vi "CRYUnflatten Stimulus Element.vi"(8 "error in (no error)":errorcluster, 11 "Unflatten Stimulus Element setup":string) -> (0 "error out":errorcluster, 1 "Stimulus Para":T1={"Name"="", "Level Out"=0.9999999999999998, "Start Freq"=6300.0, "Stop Freq"=100.0, "Steps"=19, "Cycles"=12, "Sweep type"=0, "Freq"=1000.0, "Start ampl"=0.9999999999999998, "Stop ampl"=0.9999999999999998, "sine waves"=[], "wav path"="", "Sweep time"=0.9999999999999998, "Resolution"=0, "Tone type6"=0, "fix/ratio6"=0, "Ratio6"=0, "Difference6"=0, "RatioFreq6"=0} {"Resolution" items=["R10(1/3 Oct.)", "R20(1/6 Oct.)", "R40(1/12 Oct.)", "R80(1/24 Oct.)", "User Defined, Log", "User Defined,Linear"]; "Sweep time" format="%.2f"; "Stop ampl" format="%.2f"; "Start ampl" format="%.2f"; "Freq" format="%.2f"; "sine waves"."cycles" format="%.2f"; "sine waves"."ampl" format="%.2f"; "sine waves"."freq" format="%.2f"; "Level Out" format="%.2f"}, 2 "Stimulus Default":T10={"fstepsw"={"Level(U)"=1.0, "Start Freq(Hz)"=6300.0, "Stop Freq(Hz)"=100.0, "ML val level name"="", "Use ML Val level?"=FALSE, "ML axis"=1, "Steps (#)"=19, "Cycles/step(#)"=8, "Time/step (s)"=0.01, "Step Resolution"=0, "unit"=0, "Start Freq Name"="", "Stop Freq Name"="", "Start Freq Axis"=1, "Stop Freq Axis"=1, "Start Freq Flag"="", "Stop Freq Flag"="", "Output Imp"=6300.0, "Nominal Imp"=100.0, "V on DUT"=FALSE}, "flogsw"={"Level(U)"=1.0, "Start Freq(Hz)"=100.0, "Stop Freq(Hz)"=6300.0, "Sweep Rate(s/dec)"=1.0, "Use ML Val level?"=FALSE, "ML val level name"="", "ML axis"=1, "TSR params"={"FSamp"=0.0, "FStart"=0.0, "FStop"=0.0, "NOffset"=0.0, "MStop"=0.0, "MStart"=0.0, "NHarm"=0.0, "Tsamp"=0.0, "Amplit"=0.0}, "unit"=0, "Start Freq Name"="", "Stop Freq Name"="", "Start Freq Axis"=1, "Stop Freq Axis"=1, "Start Freq Flag"="", "Stop Freq Flag"="", "Output Imp"=6300.0, "Nominal Imp"=100.0, "V on DUT"=FALSE}, "ampsw"={"Freq(Hz)"=1000.0, "Steps (#)"=19, "Cycles(#)"=12, "Use ML Val freq?"=FALSE, "ML val freq name"="", "ML axis"=1, "Start Ampl(U)"=0.5, "Stop Ampl(U)"=1.0, "unit"=0}, "wavefile"={"Level(U)"=0.0, "Wave Path"="", "ML axis"=1, "ML val level name"="", "Use ML Val level?"=FALSE, "wave info"="", "wave time"="", "Peak value4"=0.0, "RMS value4"=0.0, "wave channel"=0, "unit"=0, "Output Imp"=6300.0, "Nominal Imp"=100.0, "V on DUT"=FALSE}, "dcconn"={"dc ctrl"=0, "dcmax I"=0, "dc polar"=0, "dc ctrl"=0, "Steps (#)"=19, "Time/step (s)"=0.05, "Start Ampl(U)"=1.0, "Stop Ampl(U)"=1.0, "Level(U)"=1.0, "Step Size"=1.0}, "twotone"={"Steps (#)"=19, "Tone Type"=0, "Freq2(Hz)"=1000.0, "Time/step (s)"=0.0, "Cycles/step (#)"=12, "ML val level name"="", "Use ML Val level?"=FALSE, "Level(U) 2"=1.0, "Diff Freq(Hz)"=100.0, "ML axis 2"=1, "Diff/Ratio"=0, "Level(U)"=1.0, "Stop Freq(Hz)"=100.0, "Ratio Val"=0.8, "ML val level name 2"="", "Use ML Val level? 2"=FALSE, "ML axis"=1, "Start Freq(Hz)"=6300.0, "Step Resolution"=0, "Ratio"=0, "TabCtrl6"=enum."Master Tone", "unit 1"=0, "unit 2"=0, "Start Freq Name"="", "Stop Freq Name"="", "Start Freq Axis"=1, "Stop Freq Axis"=1, "Start Freq Flag"="", "Stop Freq Flag"=""}, "mltitone"={"Level(U)"=0.0, "Min Freq(Hz)"=0.0, "Max Freq(Hz)"=0.0, "Duration(s)"=0.0, "Freq Rounding"=FALSE, "Rounding Val"=5.0, "Profile"=0, "ML axis 2"=0, "ML val level name"="", "Use ML Val level?"=FALSE, "ML axis"=0, "Step Resolution"=0, "unit"=0, "Start Freq Name"="", "Stop Freq Name"="", "Start Freq Axis"=1, "Stop Freq Axis"=1, "Start Freq Flag"="", "Stop Freq Flag"="", "Output Imp"=6300.0, "Nominal Imp"=100.0, "V on DUT"=FALSE}, "noise"={"Noise Type"=0, "Min Freq(Hz)"=20.0, "Max Freq(Hz)"=20000.0, "Level(U)"=1.0, "Duration(s)"=1.0, "ML val level name"="", "Use ML Val level?"=FALSE, "ML axis"=1, "unit"=0, "Start Freq Name"="", "Stop Freq Name"="", "Start Freq Axis"=1, "Stop Freq Axis"=1, "Start Freq Flag"="", "Stop Freq Flag"="", "Output Imp"=6300.0, "Nominal Imp"=100.0, "V on DUT"=FALSE}, "sqwvsw"={"Level(U)"=1.0, "Duty Cycle"=0.0, "ML val level name"="", "ML axis"=1, "Start Freq(Hz)"=6300, "Stop Freq(Hz)"=100, "Use ML Val level?"=FALSE, "Steps (#)"=19, "Cycles/step (#)"=12, "Time/step (s)"=0.0, "Step Resolution"=0}, "tnbrst"={"Level(U)"=1.0, "ML val level name"="", "ML axis"=1, "Start Freq(Hz)"=6300, "Use ML Val level?"=FALSE, "Cycles/step (#)"=12, "Duration(s)"=12.0}} {"tnbrst"."Duration(s)" format="%_2f"; "tnbrst"."Level(U)" format="%_2f"; "sqwvsw"."Step Resolution" items=["R10(1/3 Oct.)", "R20(1/6 Oct.)", "R40(1/12 Oct.)", "R80(1/24 Oct.)", "User Defined, Log", "User Defined,Linear"]; "sqwvsw"."Duty Cycle" format="%_2f"; "sqwvsw"."Level(U)" format="%_2f"; "noise"."Nominal Imp" format="%.2p"; "noise"."Output Imp" format="%.2p"; "noise"."unit" items=["V  RMS", "dB re 1.0 V"]; "noise"."Duration(s)" format="%_2f"; "noise"."Level(U)" format="%_2f"; "mltitone"."Nominal Imp" format="%.2p"; "mltitone"."Output Imp" format="%.2p"; "mltitone"."unit" items=["V  RMS", "dB re 1.0 V"]; "mltitone"."Step Resolution" items=["R10(1/3 Oct.)", "R20(1/6 Oct.)", "R40(1/12 Oct.)", "R80(1/24 Oct.)", "User Defined, Log", "User Defined,Linear"]; "mltitone"."Duration(s)" format="%_2f"; "mltitone"."Level(U)" format="%_2f"; "twotone"."unit 2" items=["V  RMS", "dB re 1.0 V"]; "twotone"."unit 1" items=["V  RMS", "dB re 1.0 V"]; "twotone"."Ratio" items=["R10(1/3 Oct.)", "R20(1/6 Oct.)", "R40(1/12 Oct.)", "R80(1/24 Oct.)", "User Defined, Log", "User Defined,Linear"]; "twotone"."Step Resolution" items=["R10(1/3 Oct.)", "R20(1/6 Oct.)", "R40(1/12 Oct.)", "R80(1/24 Oct.)", "User Defined, Log", "User Defined,Linear"]; "twotone"."Ratio Val" format="%_2f"; "twotone"."Level(U)" format="%_2f"; "twotone"."Level(U) 2" format="%_2f"; "dcconn"."Step Size" format="%_3p"; "dcconn"."Level(U)" format="%_3p"; "dcconn"."Stop Ampl(U)" format="%_2f"; "dcconn"."Start Ampl(U)" format="%_2f"; "wavefile"."Nominal Imp" format="%.2p"; "wavefile"."Output Imp" format="%.2p"; "wavefile"."unit" items=["V  RMS", "dB re 1.0 V"]; "wavefile"."Level(U)" format="%_2f"; "ampsw"."unit" items=["V  RMS", "dB re 1.0 V"]; "ampsw"."Stop Ampl(U)" format="%_2f"; "ampsw"."Start Ampl(U)" format="%_2f"; "flogsw"."Nominal Imp" format="%.2p"; "flogsw"."Output Imp" format="%.2p"; "flogsw"."unit" items=["V  RMS", "dB re 1.0 V"]; "flogsw"."TSR params"."Amplit" format="%.2f"; "flogsw"."TSR params"."FStop" format="%.2f"; "flogsw"."TSR params"."FStart" format="%.2f"; "flogsw"."TSR params"."FSamp" format="%.2f"; "flogsw"."TSR params"."Tsamp" format="%.2f"; "flogsw"."TSR params"."NHarm" format="%.2f"; "flogsw"."TSR params"."MStart" format="%.2f"; "flogsw"."TSR params"."MStop" format="%.2f"; "flogsw"."TSR params"."NOffset" format="%.2f"; "flogsw"."Sweep Rate(s/dec)" format="%_2f"; "flogsw"."Level(U)" format="%_2f"; "fstepsw"."Nominal Imp" format="%.2p"; "fstepsw"."Output Imp" format="%.2p"; "fstepsw"."unit" items=["V  RMS", "dB re 1.0 V"]; "fstepsw"."Step Resolution" items=["R10(1/3 Oct.)", "R20(1/6 Oct.)", "R40(1/12 Oct.)", "R80(1/24 Oct.)", "User Defined, Log", "User Defined,Linear"]; "fstepsw"."Time/step (s)" format="%#.3p"; "fstepsw"."Cycles/step(#)" format="%.2p"; "fstepsw"."Stop Freq(Hz)" format="%.2p"; "fstepsw"."Start Freq(Hz)" format="%.2p"; "fstepsw"."Level(U)" format="%_3p"}, 3 "Header of common":T11, 4 "Type Name":string)   [LabVIEW 2013]
uses:
  Control/CRYfstepsw.ctl
  Control/CRYflogsw.ctl
  Control/CRYampsw.ctl
  Control/CRYwavefile.ctl
  Control/CRYdcconn.ctl
  Control/CRYtwotone.ctl
  Control/CRYmltitone.ctl
  Control/CRYnoise.ctl
  Typedef Control/CRYStimulus Parameter.ctl
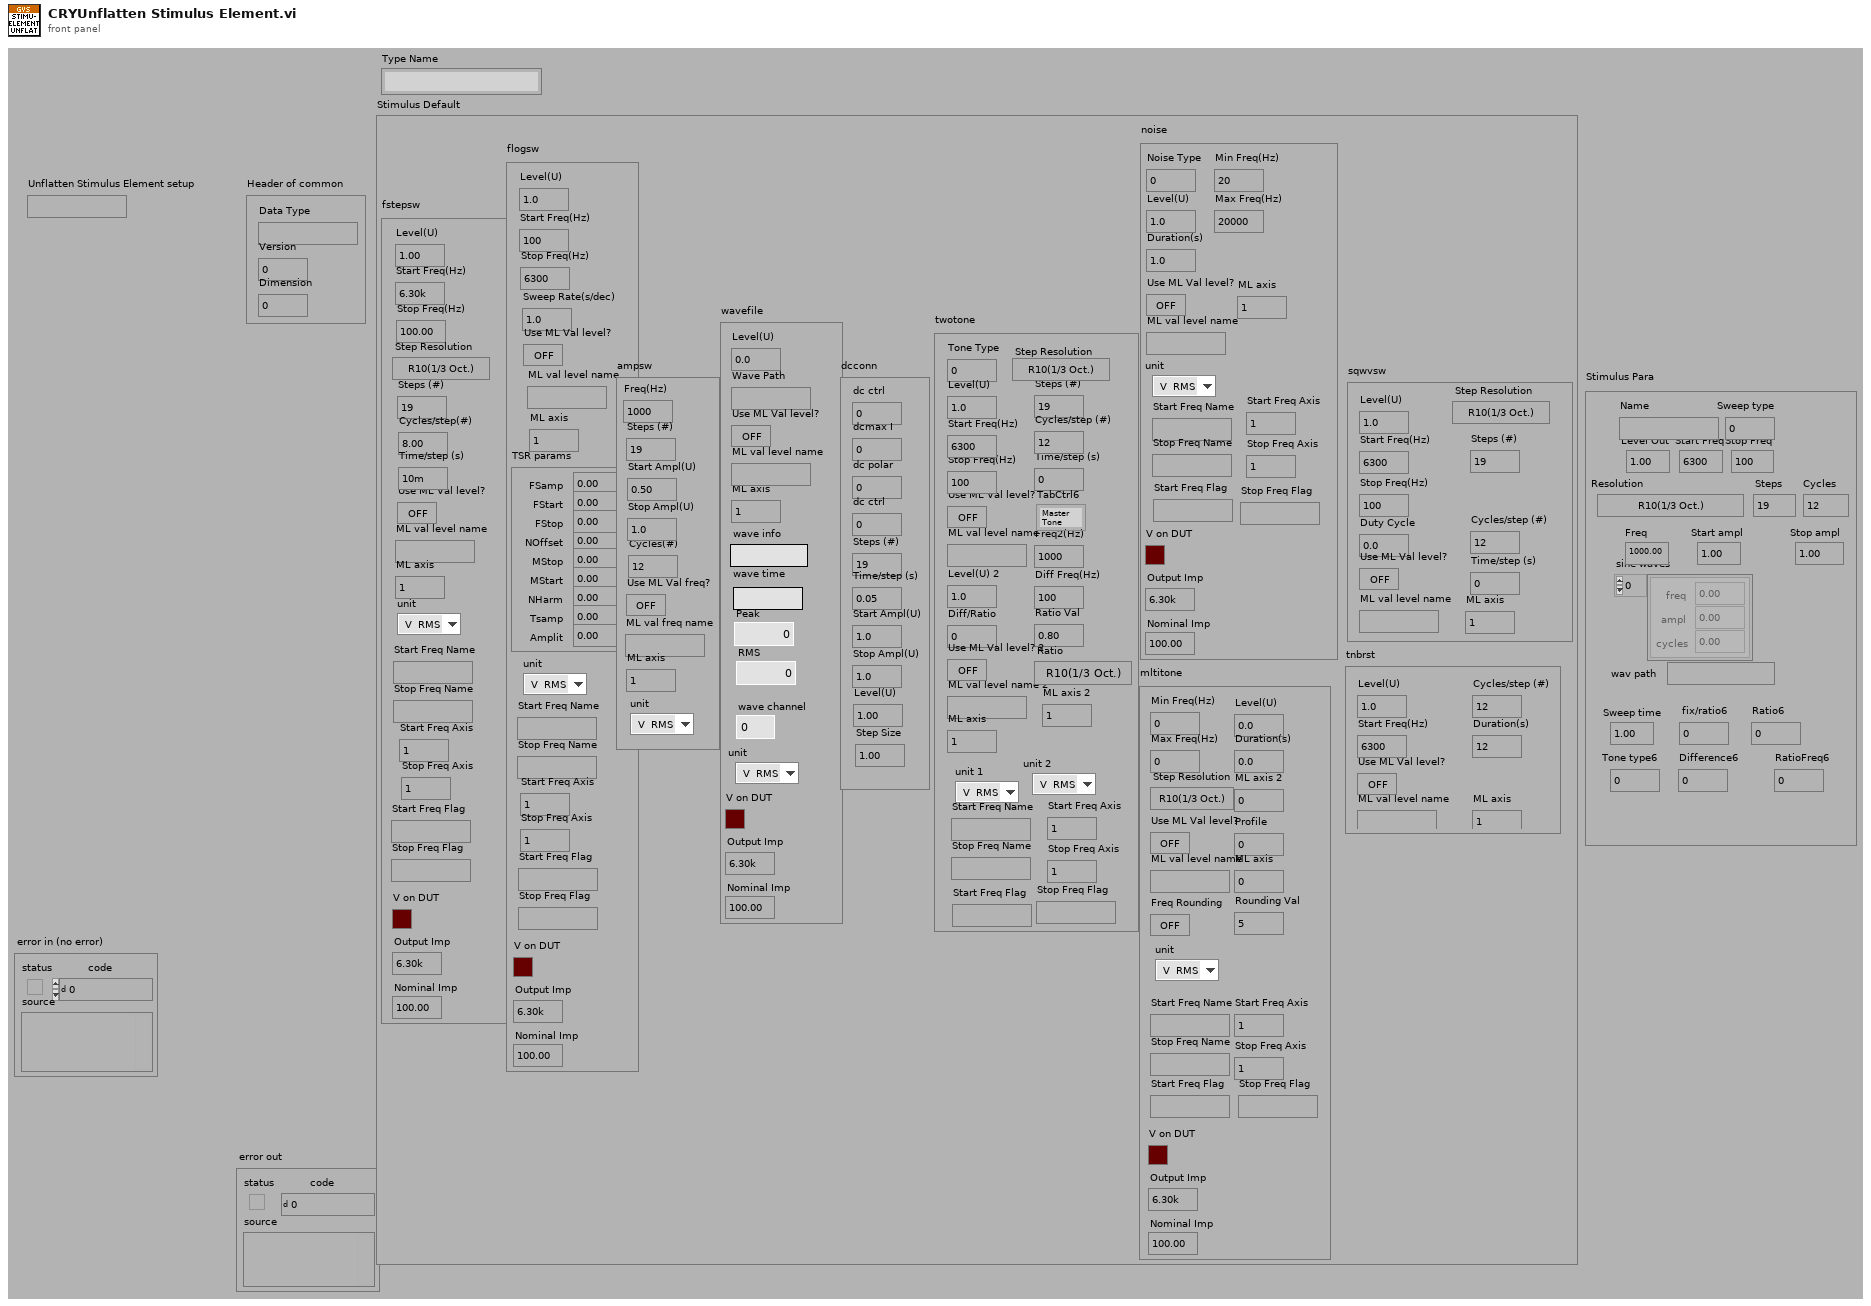
[diagram p1: front panel]
types:
  T1 = typedef "CRYStimulus Parameter.ctl" = cluster{"Name":string, "Level Out":dbl, "Start Freq":dbl, "Stop Freq":dbl, "Steps":u32, "Cycles":u32, "Sweep type":i32, "Freq":dbl, "Start ampl":dbl, "Stop ampl":dbl, "sine waves":cluster{"freq":dbl, "ampl":dbl, "cycles":dbl}[], "wav path":string, "Sweep time":dbl, "Resolution":u16, "Tone type6":u16, "fix/ratio6":u16, "Ratio6":u16, "Difference6":u32, "RatioFreq6":u32}
  T2 = typedef "CRYfstepsw.ctl" = cluster{"Level(U)":dbl, "Start Freq(Hz)":dbl, "Stop Freq(Hz)":dbl, "ML val level name":string, "Use ML Val level?":bool, "ML axis":u8, "Steps (#)":i32, "Cycles/step(#)":u32, "Time/step (s)":dbl, "Step Resolution":u16, "unit":u16, "Start Freq Name":string, "Stop Freq Name":string, "Start Freq Axis":u8, "Stop Freq Axis":u8, "Start Freq Flag":string, "Stop Freq Flag":string, "Output Imp":dbl, "Nominal Imp":dbl, "V on DUT":bool}
  T3 = typedef "CRYflogsw.ctl" = cluster{"Level(U)":dbl, "Start Freq(Hz)":dbl, "Stop Freq(Hz)":dbl, "Sweep Rate(s/dec)":dbl, "Use ML Val level?":bool, "ML val level name":string, "ML axis":u8, "TSR params":cluster{"FSamp":dbl, "FStart":dbl, "FStop":dbl, "NOffset":dbl, "MStop":dbl, "MStart":dbl, "NHarm":dbl, "Tsamp":dbl, "Amplit":dbl}, "unit":u16, "Start Freq Name":string, "Stop Freq Name":string, "Start Freq Axis":u8, "Stop Freq Axis":u8, "Start Freq Flag":string, "Stop Freq Flag":string, "Output Imp":dbl, "Nominal Imp":dbl, "V on DUT":bool}
  T4 = typedef "CRYampsw.ctl" = cluster{"Freq(Hz)":dbl, "Steps (#)":i32, "Cycles(#)":u32, "Use ML Val freq?":bool, "ML val freq name":string, "ML axis":u8, "Start Ampl(U)":dbl, "Stop Ampl(U)":dbl, "unit":u16}
  T5 = typedef "CRYwavefile.ctl" = cluster{"Level(U)":dbl, "Wave Path":string, "ML axis":u8, "ML val level name":string, "Use ML Val level?":bool, "wave info":string, "wave time":string, "Peak value4":dbl, "RMS value4":dbl, "wave channel":u16, "unit":u16, "Output Imp":dbl, "Nominal Imp":dbl, "V on DUT":bool}
  T6 = typedef "CRYdcconn.ctl" = cluster{"dc ctrl":u16, "dcmax I":u16, "dc polar":u16, "dc ctrl":u16, "Steps (#)":i32, "Time/step (s)":dbl, "Start Ampl(U)":dbl, "Stop Ampl(U)":dbl, "Level(U)":dbl, "Step Size":dbl}
  T7 = typedef "CRYtwotone.ctl" = cluster{"Steps (#)":i32, "Tone Type":u8, "Freq2(Hz)":dbl, "Time/step (s)":dbl, "Cycles/step (#)":u32, "ML val level name":string, "Use ML Val level?":bool, "Level(U) 2":dbl, "Diff Freq(Hz)":dbl, "ML axis 2":u8, "Diff/Ratio":u8, "Level(U)":dbl, "Stop Freq(Hz)":dbl, "Ratio Val":dbl, "ML val level name 2":string, "Use ML Val level? 2":bool, "ML axis":u8, "Start Freq(Hz)":dbl, "Step Resolution":u16, "Ratio":u16, "TabCtrl6":enum32{"Master Tone", "Slave Tone"}, "unit 1":u16, "unit 2":u16, "Start Freq Name":string, "Stop Freq Name":string, "Start Freq Axis":u8, "Stop Freq Axis":u8, "Start Freq Flag":string, "Stop Freq Flag":string}
  T8 = typedef "CRYmltitone.ctl" = cluster{"Level(U)":dbl, "Min Freq(Hz)":dbl, "Max Freq(Hz)":dbl, "Duration(s)":dbl, "Freq Rounding":bool, "Rounding Val":dbl, "Profile":i32, "ML axis 2":u8, "ML val level name":string, "Use ML Val level?":bool, "ML axis":u8, "Step Resolution":u16, "unit":u16, "Start Freq Name":string, "Stop Freq Name":string, "Start Freq Axis":u8, "Stop Freq Axis":u8, "Start Freq Flag":string, "Stop Freq Flag":string, "Output Imp":dbl, "Nominal Imp":dbl, "V on DUT":bool}
  T9 = typedef "CRYnoise.ctl" = cluster{"Noise Type":u8, "Min Freq(Hz)":dbl, "Max Freq(Hz)":dbl, "Level(U)":dbl, "Duration(s)":dbl, "ML val level name":string, "Use ML Val level?":bool, "ML axis":u8, "unit":u16, "Start Freq Name":string, "Stop Freq Name":string, "Start Freq Axis":u8, "Stop Freq Axis":u8, "Start Freq Flag":string, "Stop Freq Flag":string, "Output Imp":dbl, "Nominal Imp":dbl, "V on DUT":bool}
  T10 = cluster{"fstepsw":T2, "flogsw":T3, "ampsw":T4, "wavefile":T5, "dcconn":T6, "twotone":T7, "mltitone":T8, "noise":T9, "sqwvsw":cluster{"Level(U)":dbl, "Duty Cycle":dbl, "ML val level name":string, "ML axis":u8, "Start Freq(Hz)":u32, "Stop Freq(Hz)":u32, "Use ML Val level?":bool, "Steps (#)":u32, "Cycles/step (#)":u32, "Time/step (s)":dbl, "Step Resolution":u16}, "tnbrst":cluster{"Level(U)":dbl, "ML val level name":string, "ML axis":u8, "Start Freq(Hz)":u32, "Use ML Val level?":bool, "Cycles/step (#)":u32, "Duration(s)":dbl}}
  T11 = cluster{"Data Type":string, "Version":u16, "Dimension":u8}
  T12 = cluster{"Level(U)":dbl, "Start Freq(Hz)":dbl, "Stop Freq(Hz)":dbl, "ML val level name":string, "Use ML Val level?":bool, "ML axis":u8, "Steps (#)":i32, "Cycles/step(#)":u32, "Time/step (s)":dbl, "Step Resolution":u16}
  T13 = cluster{"Level(U)":dbl, "Start Freq(Hz)":dbl, "Stop Freq(Hz)":dbl, "Sweep Rate(s/dec)":dbl, "Use ML Val level?":bool, "ML val level name":string, "ML axis":u8, "TSR params":cluster{"FSamp":dbl, "FStart":dbl, "FStop":dbl, "NOffset":dbl, "MStop":dbl, "MStart":dbl, "NHarm":dbl, "Tsamp":dbl, "Amplit":dbl}}
  T14 = cluster{"Freq(Hz)":dbl, "Steps (#)":i32, "Cycles(#)":u32, "Use ML Val freq?":bool, "ML val freq name":string, "ML axis":u8, "Start Ampl(U)":dbl, "Stop Ampl(U)":dbl}
  T15 = cluster{"Level(U)":dbl, "Wave Path":string, "ML axis":u8, "ML val level name":string, "Use ML Val level?":bool, "wave info":string, "wave time":string, "Peak value4":dbl, "RMS value4":dbl}
  T16 = cluster{"dc ctrl":u16, "dcmax I":u16, "dc polar":u16, "dc ctrl":u16, "Steps (#)":i32, "Time/step (s)":dbl, "Start Ampl(U)":dbl, "Stop Ampl(U)":dbl, "Level(U)":dbl, "Step Size":dbl}
  T17 = cluster{"Steps (#)":i32, "Tone Type":u8, "Freq2(Hz)":dbl, "Time/step (s)":dbl, "Cycles/step (#)":u32, "ML val level name":string, "Use ML Val level?":bool, "Level(U) 2":dbl, "Diff Freq(Hz)":dbl, "ML axis 2":u8, "Diff/Ratio":u8, "Level(U)":dbl, "Stop Freq(Hz)":dbl, "Ratio Val":dbl, "ML val level name 2":string, "Use ML Val level? 2":bool, "ML axis":u8, "Start Freq(Hz)":dbl, "Step Resolution":u16, "Ratio":u16, "TabCtrl6":enum32{"Master Tone", "Slave Tone"}}
  T18 = cluster{"Noise Type":u8, "Min Freq(Hz)":dbl, "Max Freq(Hz)":dbl, "Level(U)":dbl, "Duration(s)":dbl, "ML val level name":string, "Use ML Val level?":bool, "ML axis":u8}
  T19 = cluster{"Level(U)":dbl, "Min Freq(Hz)":dbl, "Max Freq(Hz)":dbl, "Duration(s)":dbl, "Freq Rounding":bool, "Rounding Val":dbl, "Profile":i32, "ML axis 2":u8, "ML val level name":string, "Use ML Val level?":bool, "ML axis":u8, "Step Resolution":u16}
  T20 = cluster{"Level(U)":dbl, "Wave Path":string, "ML axis":u8, "ML val level name":string, "Use ML Val level?":bool, "wave info":string, "wave time":string, "Peak value4":dbl, "RMS value4":dbl, "wave channel":u16}
  T21 = cluster{"Level(U)":dbl, "Start Freq(Hz)":dbl, "Stop Freq(Hz)":dbl, "ML val level name":string, "Use ML Val level?":bool, "ML axis":u8, "Steps (#)":i32, "Cycles/step(#)":u32, "Time/step (s)":dbl, "Step Resolution":u16, "unit":u16}
  T22 = cluster{"Level(U)":dbl, "Start Freq(Hz)":dbl, "Stop Freq(Hz)":dbl, "Sweep Rate(s/dec)":dbl, "Use ML Val level?":bool, "ML val level name":string, "ML axis":u8, "TSR params":cluster{"FSamp":dbl, "FStart":dbl, "FStop":dbl, "NOffset":dbl, "MStop":dbl, "MStart":dbl, "NHarm":dbl, "Tsamp":dbl, "Amplit":dbl}, "unit":u16}
  T23 = cluster{"Freq(Hz)":dbl, "Steps (#)":i32, "Cycles(#)":u32, "Use ML Val freq?":bool, "ML val freq name":string, "ML axis":u8, "Start Ampl(U)":dbl, "Stop Ampl(U)":dbl, "unit":u16}
  T24 = cluster{"Level(U)":dbl, "Wave Path":string, "ML axis":u8, "ML val level name":string, "Use ML Val level?":bool, "wave info":string, "wave time":string, "Peak value4":dbl, "RMS value4":dbl, "wave channel":u16, "unit":u16}
  T25 = cluster{"Steps (#)":i32, "Tone Type":u8, "Freq2(Hz)":dbl, "Time/step (s)":dbl, "Cycles/step (#)":u32, "ML val level name":string, "Use ML Val level?":bool, "Level(U) 2":dbl, "Diff Freq(Hz)":dbl, "ML axis 2":u8, "Diff/Ratio":u8, "Level(U)":dbl, "Stop Freq(Hz)":dbl, "Ratio Val":dbl, "ML val level name 2":string, "Use ML Val level? 2":bool, "ML axis":u8, "Start Freq(Hz)":dbl, "Step Resolution":u16, "Ratio":u16, "TabCtrl6":enum32{"Master Tone", "Slave Tone"}, "unit 1":u16, "unit 2":u16}
  T26 = cluster{"Noise Type":u8, "Min Freq(Hz)":dbl, "Max Freq(Hz)":dbl, "Level(U)":dbl, "Duration(s)":dbl, "ML val level name":string, "Use ML Val level?":bool, "ML axis":u8, "unit":u16}
  T27 = cluster{"Level(U)":dbl, "Min Freq(Hz)":dbl, "Max Freq(Hz)":dbl, "Duration(s)":dbl, "Freq Rounding":bool, "Rounding Val":dbl, "Profile":i32, "ML axis 2":u8, "ML val level name":string, "Use ML Val level?":bool, "ML axis":u8, "Step Resolution":u16, "unit":u16}
  T28 = cluster{"unsigned byte array[0]":u8, "unsigned byte array[1]":u8, "unsigned byte array[2]":u8}
  T29 = cluster{"FSamp":dbl, "FStart":dbl, "FStop":dbl, "NOffset":dbl, "MStop":dbl, "MStart":dbl, "NHarm":dbl, "Tsamp":dbl, "Amplit":dbl}
  T30 = cluster{"Level(U)":dbl, "Start Freq(Hz)":dbl, "Stop Freq(Hz)":dbl, "ML val level name":string, "Use ML Val level?":bool, "ML axis":u8, "Steps (#)":i32, "Cycles/step(#)":u32, "Time/step (s)":dbl, "Step Resolution":u16, "unit":u16, "Start Freq Name":string, "Stop Freq Name":string, "Start Freq Axis":u8, "Stop Freq Axis":u8, "Start Freq Flag":string, "Stop Freq Flag":string}
  T31 = cluster{"Level(U)":dbl, "Start Freq(Hz)":dbl, "Stop Freq(Hz)":dbl, "Sweep Rate(s/dec)":dbl, "Use ML Val level?":bool, "ML val level name":string, "ML axis":u8, "TSR params":cluster{"FSamp":dbl, "FStart":dbl, "FStop":dbl, "NOffset":dbl, "MStop":dbl, "MStart":dbl, "NHarm":dbl, "Tsamp":dbl, "Amplit":dbl}, "unit":u16, "Start Freq Name":string, "Stop Freq Name":string, "Start Freq Axis":u8, "Stop Freq Axis":u8, "Start Freq Flag":string, "Stop Freq Flag":string}
  T32 = cluster{"Steps (#)":i32, "Tone Type":u8, "Freq2(Hz)":dbl, "Time/step (s)":dbl, "Cycles/step (#)":u32, "ML val level name":string, "Use ML Val level?":bool, "Level(U) 2":dbl, "Diff Freq(Hz)":dbl, "ML axis 2":u8, "Diff/Ratio":u8, "Level(U)":dbl, "Stop Freq(Hz)":dbl, "Ratio Val":dbl, "ML val level name 2":string, "Use ML Val level? 2":bool, "ML axis":u8, "Start Freq(Hz)":dbl, "Step Resolution":u16, "Ratio":u16, "TabCtrl6":enum32{"Master Tone", "Slave Tone"}, "unit 1":u16, "unit 2":u16, "Start Freq Name":string, "Stop Freq Name":string, "Start Freq Axis":u8, "Stop Freq Axis":u8, "Start Freq Flag":string, "Stop Freq Flag":string}
  T33 = cluster{"Noise Type":u8, "Min Freq(Hz)":dbl, "Max Freq(Hz)":dbl, "Level(U)":dbl, "Duration(s)":dbl, "ML val level name":string, "Use ML Val level?":bool, "ML axis":u8, "unit":u16, "Start Freq Name":string, "Stop Freq Name":string, "Start Freq Axis":u8, "Stop Freq Axis":u8, "Start Freq Flag":string, "Stop Freq Flag":string}
  T34 = cluster{"Level(U)":dbl, "Min Freq(Hz)":dbl, "Max Freq(Hz)":dbl, "Duration(s)":dbl, "Freq Rounding":bool, "Rounding Val":dbl, "Profile":i32, "ML axis 2":u8, "ML val level name":string, "Use ML Val level?":bool, "ML axis":u8, "Step Resolution":u16, "unit":u16, "Start Freq Name":string, "Stop Freq Name":string, "Start Freq Axis":u8, "Stop Freq Axis":u8, "Start Freq Flag":string, "Stop Freq Flag":string}
  T35 = cluster{"Unflatten Stimulus Element setup":string, u16, "unsigned byte array[2]":u8}
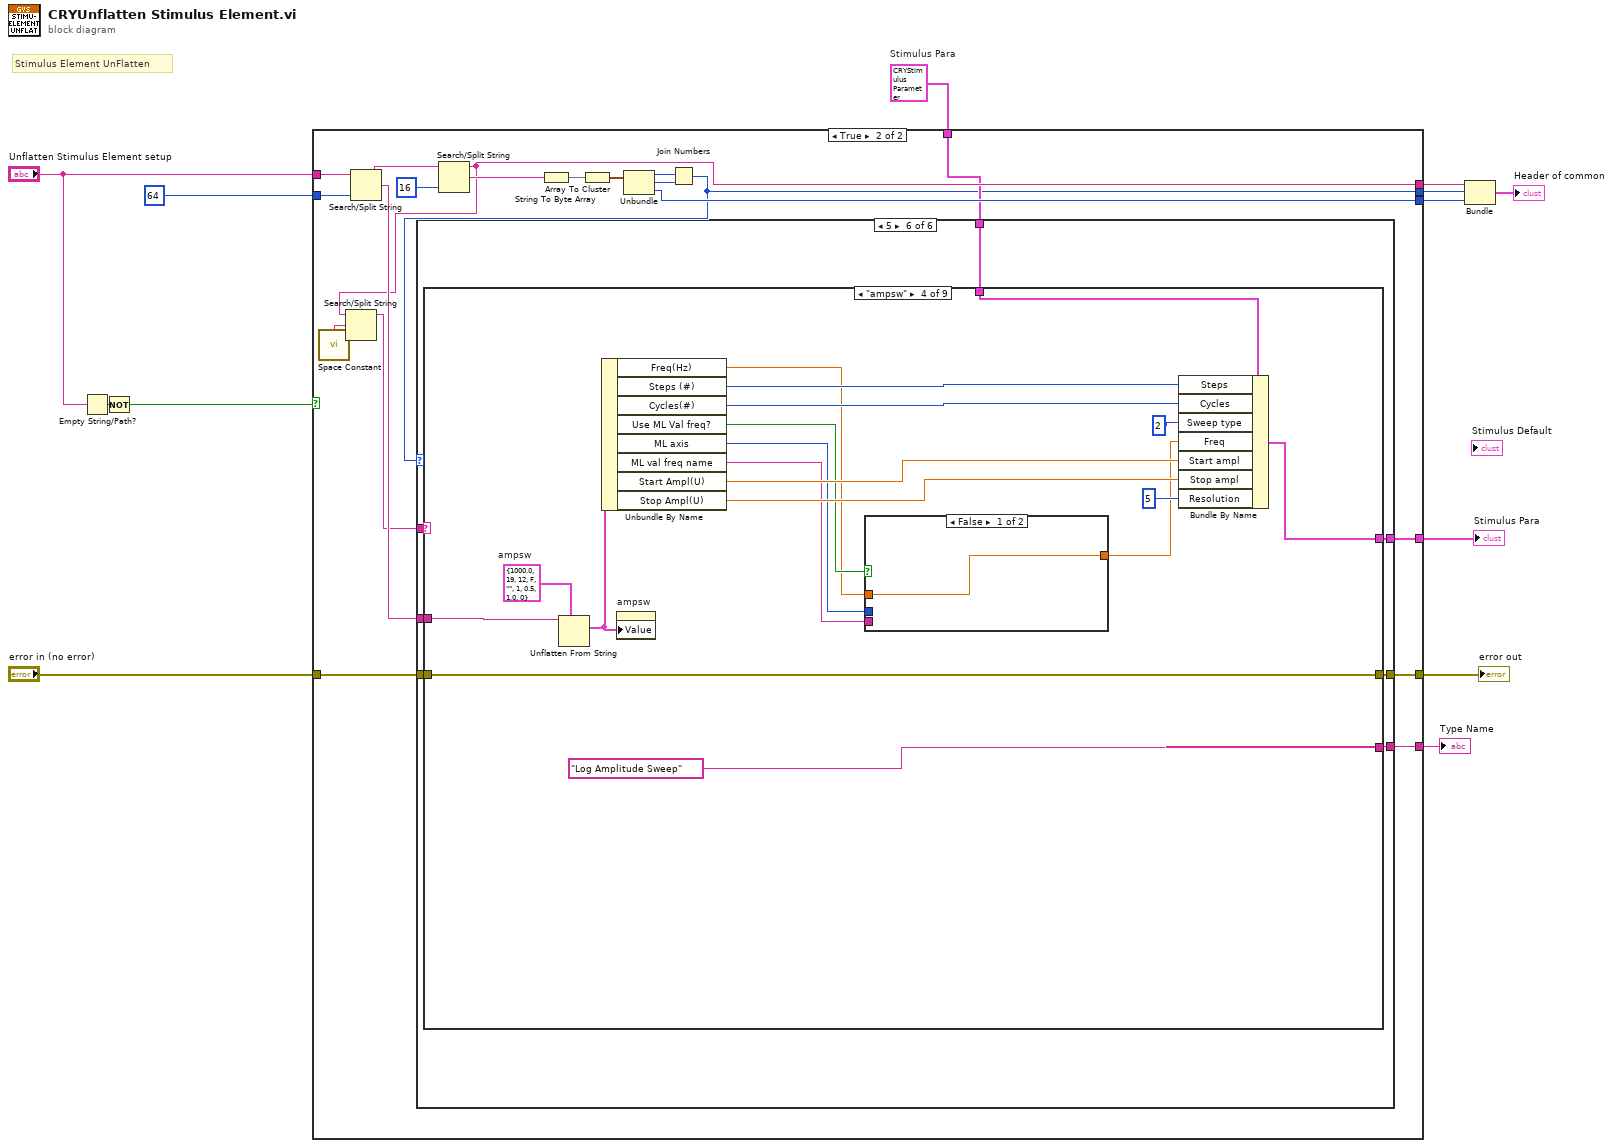
[diagram p0: block diagram]
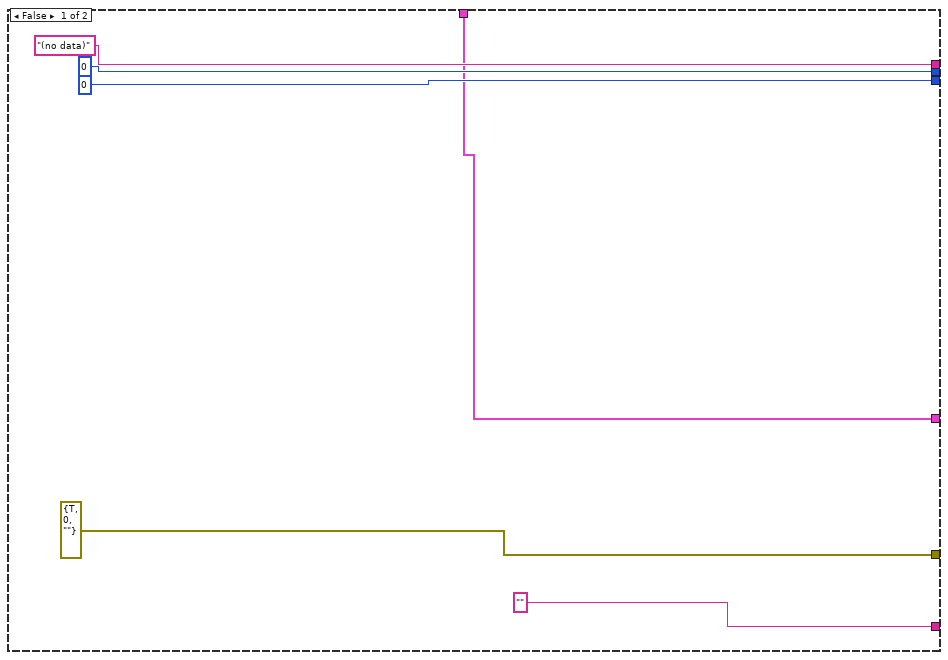
[diagram p2: hidden frame]
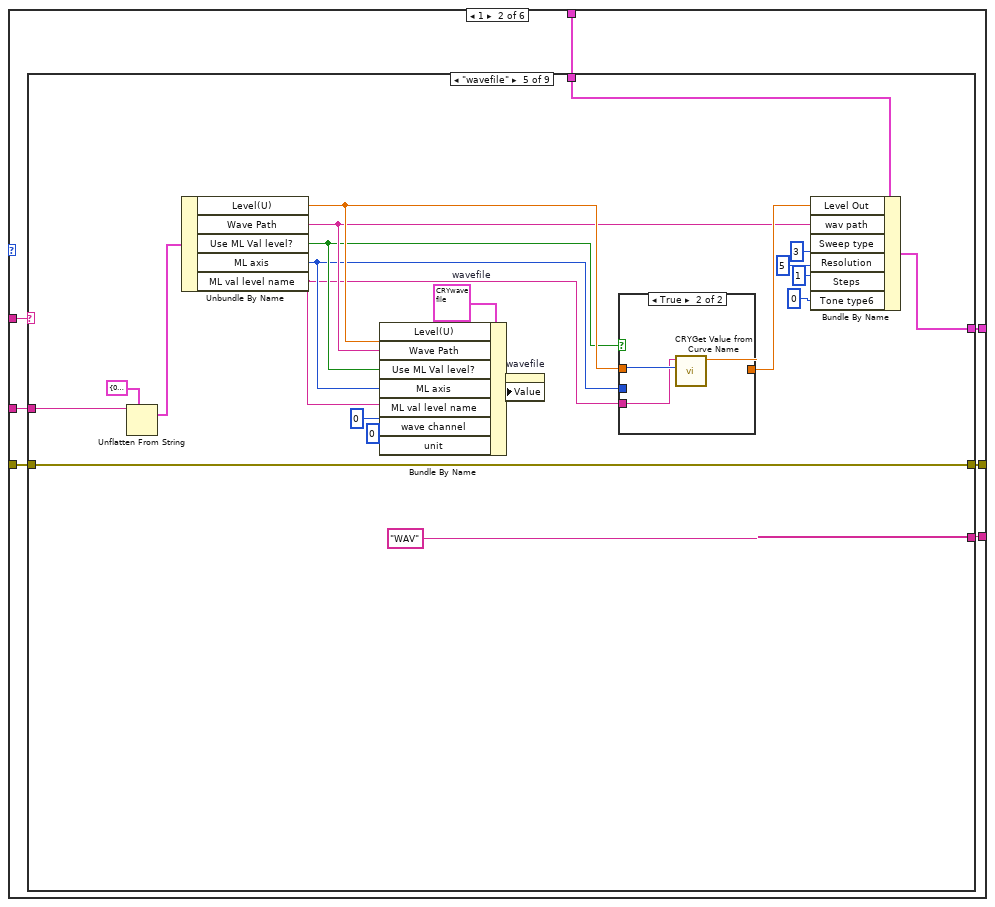
[diagram p4: hidden frame]
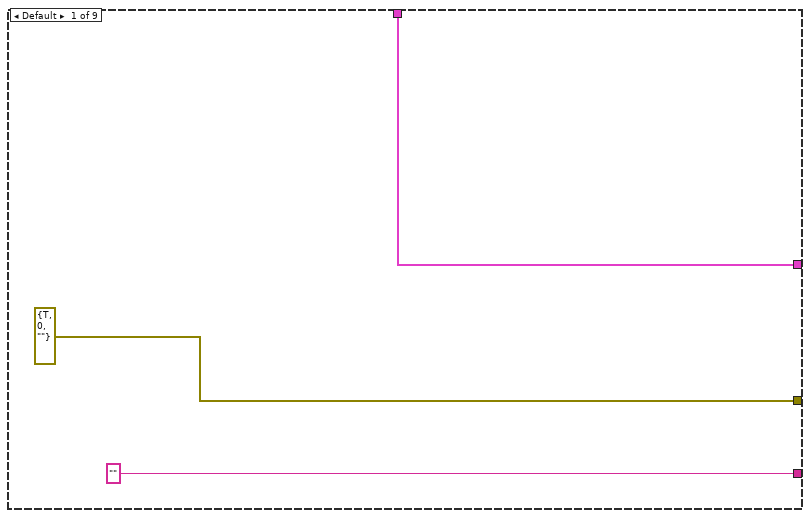
[diagram p5: hidden frame]
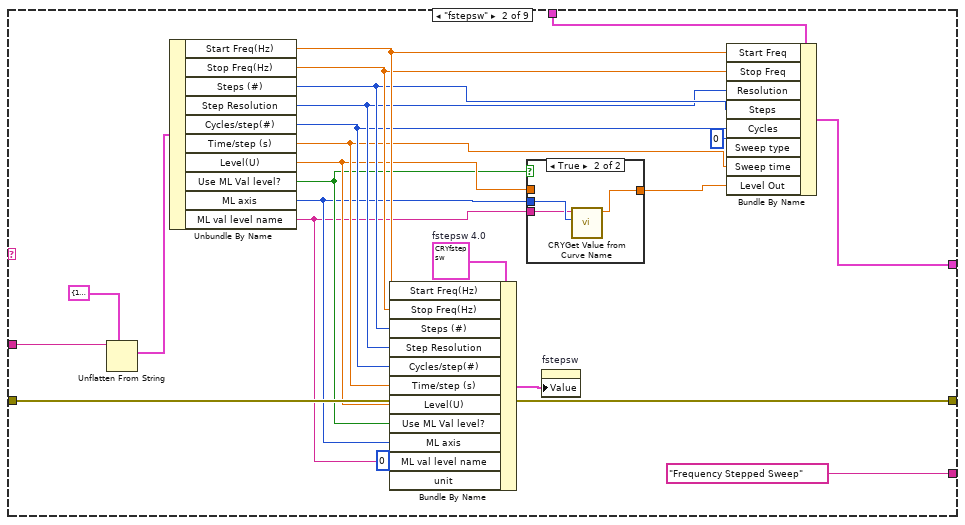
[diagram p6: hidden frame]
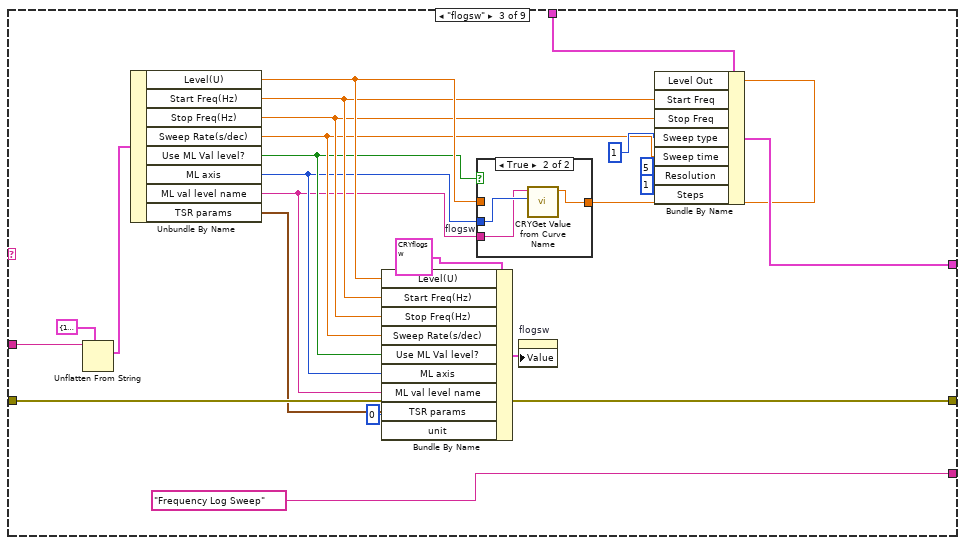
[diagram p8: hidden frame]
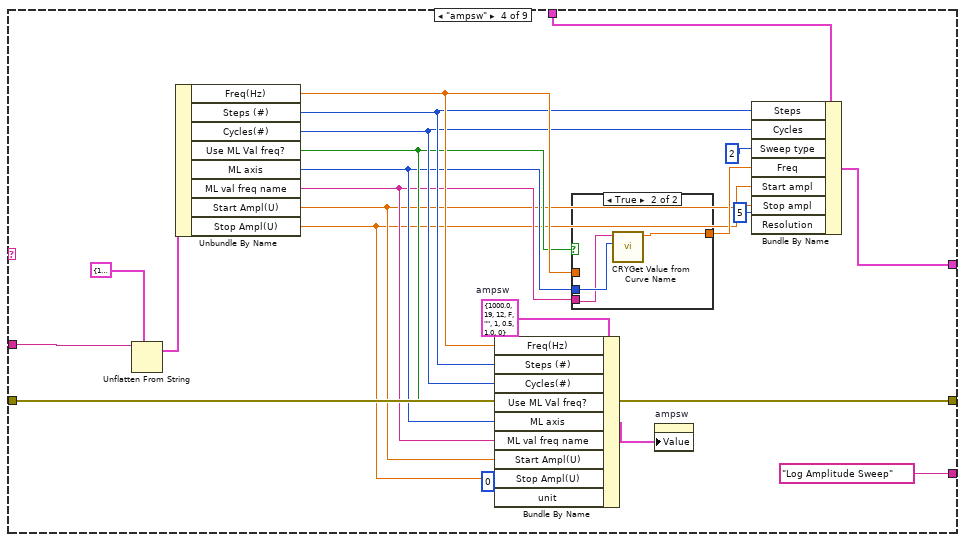
[diagram p10: hidden frame]
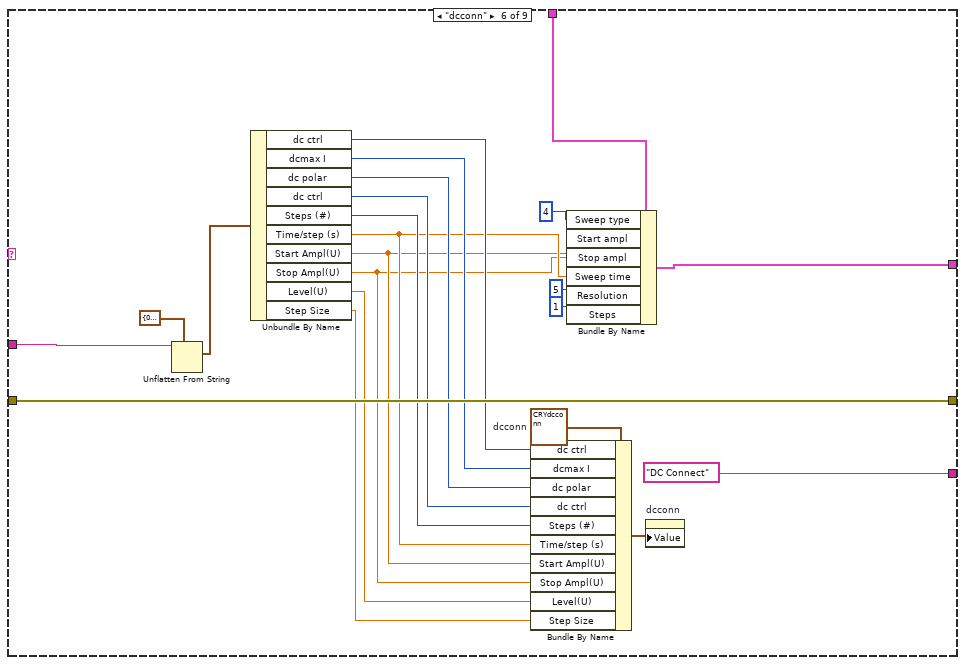
[diagram p13: hidden frame]
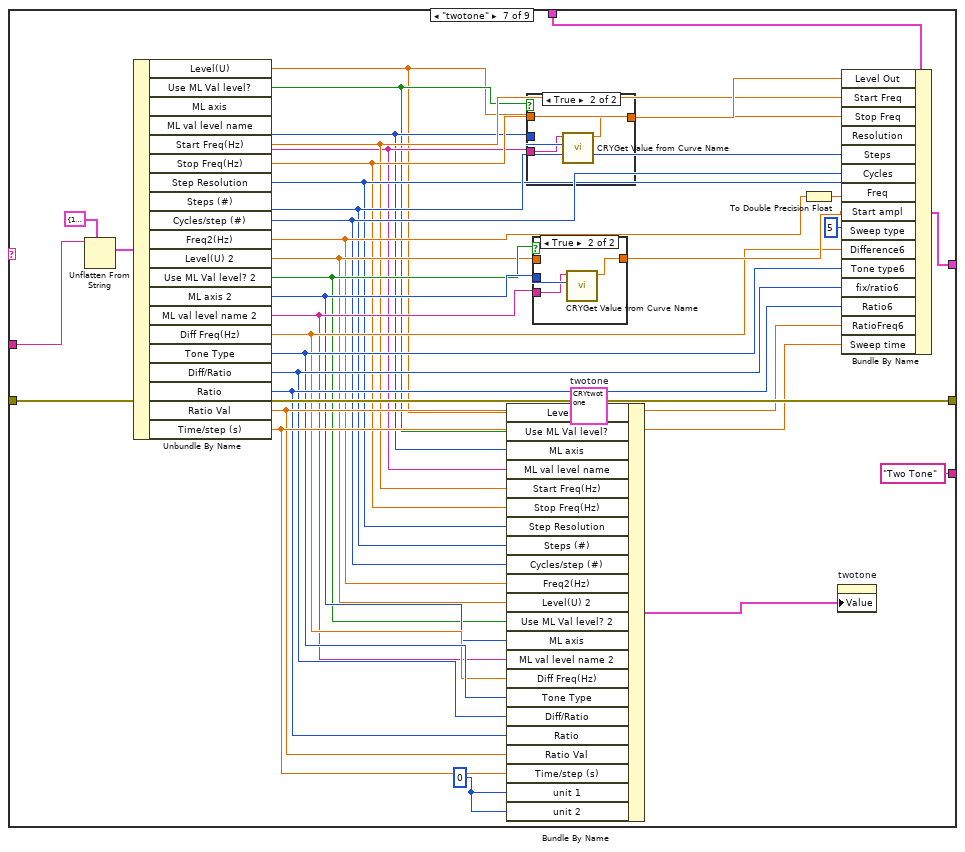
[diagram p14: hidden frame]
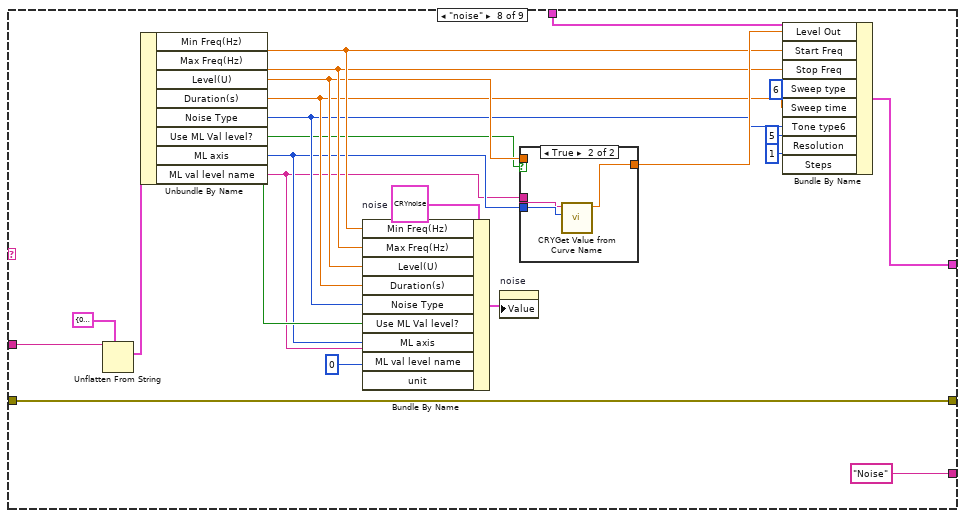
[diagram p17: hidden frame]
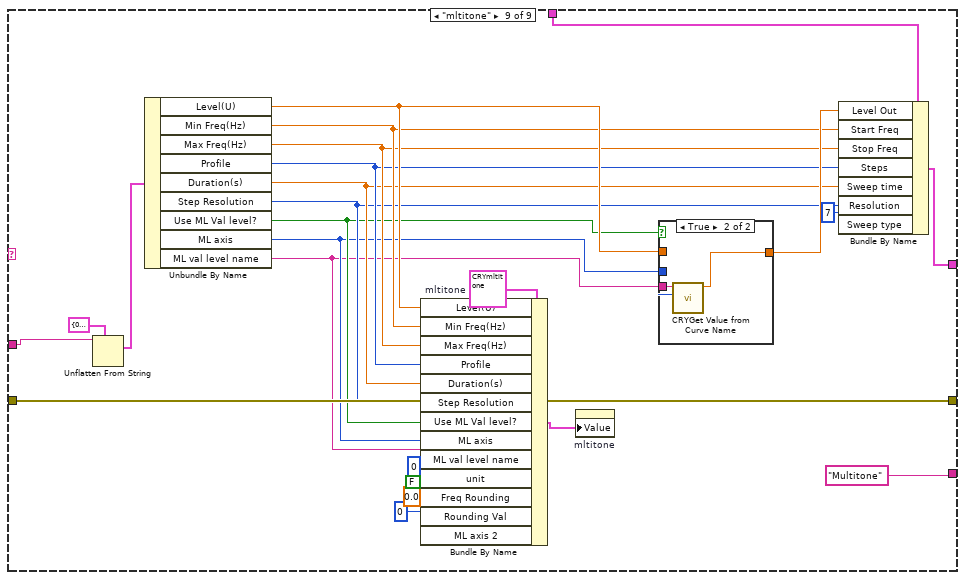
[diagram p19: hidden frame]
diagram:
  w2 = T1 {"Name"="", "Level Out"=0.9999999999999998, "Start Freq"=6300.0, "Stop Freq"=100.0, "Steps"=19, "Cycles"=12, "Sweep type"=0, "Freq"=1000.0, "Start ampl"=0.9999999999999998, "Stop ampl"=0.9999999999999998, "sine waves"=[], "wav path"="", "Sweep time"=0.9999999999999998, "Resolution"=0, "Tone type6"=0, "fix/ratio6"=0, "Ratio6"=0, "Difference6"=0, "RatioFreq6"=0}  # Stimulus Para
  # "Stimulus Element UnFlatten"
  n1 = Empty String/Path?(string/path="Unflatten Stimulus Element setup") -> (empty?=w12:bool)
  n2 = Not(x=w12) -> (.not. x?=w4:bool)
  n3 = case shown="True" w4 {
    tunnel: "Unflatten Stimulus Element setup" -> [_ w30]
    tunnel: 64 -> [_ w39]
    tunnel: [u16 0 w20] -> w9
    tunnel: [u8 0 w31] -> w8
    tunnel: ["(no data)" w24] -> w7
    tunnel: [errorcluster {"status"=TRUE, "code"=0, "source"=""} ("error in (no error)") w28] -> w6
    tunnel: "error in (no error)" -> [_ w27]
    tunnel: [w14 w26] -> w1
    tunnel: ["" w22] -> w3
    tunnel: w2 -> [w14 w21]
    frame False {
    }
    frame True {
      n4 = call <vilib>:"Space Constant.vi"() -> ("String"=w25:string)
      n5 = Search/Split String(string=w30, offset (0)=w39) -> (substring before match=w38:string, match + rest of string=w29:string)  [unwired: 2 out]
      n6 = Search/Split String(string=w38, offset (0)=16 ("length (rest)")) -> (substring before match=w24:string, match + rest of string=w36:string)  [unwired: 2 out]
      n7 = Search/Split String(string=w24, search string/char (-)=w25) -> (substring before match=w23:string)  [unwired: 3 out]
      n8 = String To Byte Array(string=w36) -> (unsigned byte array=w35:u8[])
      n9 = Array To Cluster(array=w35) -> (cluster=w34:T28)
      n10 = Unbundle(w34) -> ("unsigned byte array[0]"=w33:u8, "unsigned byte array[1]"=w32:u8, "unsigned byte array[2]"=w31:u8)
      n11 = Join Numbers(hi=w33, lo=w32) -> ((hi.lo)=w20:u16)
      n12 = case shown="5" w20 {
        tunnel: w29 -> [_ w48 w278 w507 w737 w967]
        tunnel: [w40 w47 w277 w506 w736 w966] -> w28
        tunnel: w27 -> [w40 w46 w276 w505 w735 w965]
        tunnel: [w41 w45 w275 w504 w734 w964] -> w26
        tunnel: w23 -> [_ w44 w274 w503 w733 w963]
        tunnel: [_ w43 w273 w502 w732 w962] -> w22
        tunnel: w21 -> [w41 w42 w272 w501 w731 w961]
        frame Default {
        }
        frame 1 {
          n13 = case shown="\"wavefile\"" w44 {
            tunnel: w48 -> [_ w73 w99 w124 w148 w174 w208 w238 w266]
            tunnel: [errorcluster {"status"=TRUE, "code"=0, "source"=""} ("error in (no error)") w72 w98 w123 w149 w175 w209 w239 w267] -> w47
            tunnel: w46 -> [_ w72 w98 w123 w149 w175 w209 w239 w267]
            tunnel: w42 -> [w50 w68 w96 w121 w145 w173 w207 w237 w264]
            tunnel: [w50 w70 w94 w119 w146 w172 w206 w235 w263] -> w45
            tunnel: ["" "Frequency Stepped Sweep" "Frequency Log Sweep" "Log Amplitude Sweep" "WAV" "DC Connect" "Two Tone" "Noise" "Multitone"] -> w43
            frame Default {
            }
            frame "fstepsw" {
              w53 = T2 {"Level(U)"=0.7071067811865476, "Start Freq(Hz)"=20000.0, "Stop Freq(Hz)"=20.0, "ML val level name"="Calibration sens-out Left", "Use ML Val level?"=FALSE, "ML axis"=0, "Steps (#)"=31, "Cycles/step(#)"=20, "Time/step (s)"=0.01, "Step Resolution"=0, "unit"=0, "Start Freq Name"="Calibration sens-out Left", "Stop Freq Name"="Calibration sens-out Left", "Start Freq Axis"=0, "Stop Freq Axis"=0, "Start Freq Flag"="", "Stop Freq Flag"="", "Output Imp"=0.0, "Nominal Imp"=0.0, "V on DUT"=FALSE}  # fstepsw 4.0
              n14 = Unflatten From String(type=T12 {"Level(U)"=1.0, "Start Freq(Hz)"=6300.0, "Stop Freq(Hz)"=100.0, "ML val level name"="", "Use ML Val level?"=FALSE, "ML axis"=1, "Steps (#)"=19, "Cycles/step(#)"=8, "Time/step (s)"=0.01, "Step Resolution"=0} ("fstepsw"), binary string=w73) -> (value=w69:T12)  [unwired: 1 in, 4 out]
              n15 = Unbundle By Name(w69) -> ("Start Freq(Hz)"=w65:dbl, "Stop Freq(Hz)"=w64:dbl, "Steps (#)"=w63:i32, "Step Resolution"=w62:u16, "Cycles/step(#)"=w61:u32, "Time/step (s)"=w60:dbl, "Level(U)"=w59:dbl, "Use ML Val level?"=w58:bool, "ML axis"=w57:u8, "ML val level name"=w56:string)
              n16 = Bundle By Name(cluster=w53, "Start Freq(Hz)"=w65, "Stop Freq(Hz)"=w64, "Steps (#)"=w63, "Step Resolution"=w62, "Cycles/step(#)"=w61, "Time/step (s)"=w60, "Level(U)"=w59, "Use ML Val level?"=w58, "ML axis"=w57, "ML val level name"=w56, "unit"=u16 0) -> (w55:T2)
              n17 = case shown="True" w58 {
                tunnel: w57 -> [_ w77]
                tunnel: w59 -> [w74 _]
                tunnel: [w74 w75] -> w66
                tunnel: w56 -> [_ w76]
                frame False {
                }
                frame True {
                  n18 = call "CRYGet Value from Curve Name.vi"("ML axis"=w77, "Level Name"=w76) -> ("Linear Value"=w75:dbl)  [unwired: 9 in]
                }
              }
              n19 = property on="fstepsw" class="Clust (strict)"("Value"=w55) -> ()  [unwired: 2 in, 2 out]
              n20 = Bundle By Name(cluster=w68, "Start Freq"=w65, "Stop Freq"=w64, "Resolution"=w62, "Steps"=w63, "Cycles"=w61, "Sweep type"=0, "Sweep time"=w60, "Level Out"=w66) -> (w70:T1)
            }
            frame "flogsw" {
              w79 = T3 {"Level(U)"=1.0, "Start Freq(Hz)"=100.0, "Stop Freq(Hz)"=6300.0, "Sweep Rate(s/dec)"=1.0, "Use ML Val level?"=FALSE, "ML val level name"="", "ML axis"=1, "TSR params"={"FSamp"=0.0, "FStart"=0.0, "FStop"=0.0, "NOffset"=0.0, "MStop"=0.0, "MStart"=0.0, "NHarm"=0.0, "Tsamp"=0.0, "Amplit"=0.0}, "unit"=0, "Start Freq Name"="Calibration sens-out Left", "Stop Freq Name"="Calibration sens-out Left", "Start Freq Axis"=0, "Stop Freq Axis"=0, "Start Freq Flag"="", "Stop Freq Flag"="", "Output Imp"=0.0, "Nominal Imp"=0.0, "V on DUT"=FALSE}  # flogsw
              n21 = Unflatten From String(type=T13 {"Level(U)"=1.0, "Start Freq(Hz)"=100.0, "Stop Freq(Hz)"=6300.0, "Sweep Rate(s/dec)"=1.0, "Use ML Val level?"=FALSE, "ML val level name"="", "ML axis"=1, "TSR params"={"FSamp"=0.0, "FStart"=0.0, "FStop"=0.0, "NOffset"=0.0, "MStop"=0.0, "MStart"=0.0, "NHarm"=0.0, "Tsamp"=0.0, "Amplit"=0.0}} ("flogsw"), binary string=w99) -> (value=w97:T13)  [unwired: 1 in, 4 out]
              n22 = Unbundle By Name(w97) -> ("Level(U)"=w89:dbl, "Start Freq(Hz)"=w88:dbl, "Stop Freq(Hz)"=w87:dbl, "Sweep Rate(s/dec)"=w86:dbl, "Use ML Val level?"=w85:bool, "ML axis"=w84:u8, "ML val level name"=w83:string, "TSR params"=w82:T29)
              n23 = Bundle By Name(cluster=w79, "Level(U)"=w89, "Start Freq(Hz)"=w88, "Stop Freq(Hz)"=w87, "Sweep Rate(s/dec)"=w86, "Use ML Val level?"=w85, "ML axis"=w84, "ML val level name"=w83, "TSR params"=w82, "unit"=u16 0) -> (w80:T3)
              n24 = case shown="True" w85 {
                tunnel: w84 -> [_ w103]
                tunnel: w89 -> [w100 _]
                tunnel: [w100 w101] -> w90
                tunnel: w83 -> [_ w102]
                frame False {
                }
                frame True {
                  n25 = call "CRYGet Value from Curve Name.vi"("ML axis"=w103, "Level Name"=w102) -> ("Linear Value"=w101:dbl)  [unwired: 9 in]
                }
              }
              n26 = property on="flogsw" class="Clust (strict)"("Value"=w80) -> ()  [unwired: 2 in, 2 out]
              n27 = Bundle By Name(cluster=w96, "Level Out"=w90, "Start Freq"=w88, "Stop Freq"=w87, "Sweep type"=1, "Sweep time"=w86, "Resolution"=u16 5, "Steps"=u32 1) -> (w94:T1)
            }
            frame "ampsw" {
              w105 = T4 {"Freq(Hz)"=1000.0, "Steps (#)"=19, "Cycles(#)"=12, "Use ML Val freq?"=FALSE, "ML val freq name"="", "ML axis"=1, "Start Ampl(U)"=0.5, "Stop Ampl(U)"=1.0, "unit"=0}  # ampsw
              n28 = Unflatten From String(type=T14 {"Freq(Hz)"=1000.0, "Steps (#)"=19, "Cycles(#)"=12, "Use ML Val freq?"=FALSE, "ML val freq name"="", "ML axis"=1, "Start Ampl(U)"=0.5, "Stop Ampl(U)"=1.0} ("ampsw"), binary string=w124) -> (value=w122:T14)  [unwired: 1 in, 4 out]
              n29 = Unbundle By Name(w122) -> ("Freq(Hz)"=w115:dbl, "Steps (#)"=w114:i32, "Cycles(#)"=w113:u32, "Use ML Val freq?"=w112:bool, "ML axis"=w111:u8, "ML val freq name"=w110:string, "Start Ampl(U)"=w109:dbl, "Stop Ampl(U)"=w108:dbl)
              n30 = Bundle By Name(cluster=w105, "Freq(Hz)"=w115, "Steps (#)"=w114, "Cycles(#)"=w113, "Use ML Val freq?"=w112, "ML axis"=w111, "ML val freq name"=w110, "Start Ampl(U)"=w109, "Stop Ampl(U)"=w108, "unit"=u16 0) -> (w106:T4)
              n31 = case shown="True" w112 {
                tunnel: w111 -> [_ w128]
                tunnel: w115 -> [w125 _]
                tunnel: [w125 w126] -> w116
                tunnel: w110 -> [_ w127]
                frame False {
                }
                frame True {
                  n32 = call "CRYGet Value from Curve Name.vi"("ML axis"=w128, "Level Name"=w127) -> ("Linear Value"=w126:dbl)  [unwired: 9 in]
                }
              }
              n33 = property on="ampsw" class="Clust (strict)"("Value"=w106) -> ()  [unwired: 2 in, 2 out]
              n34 = Bundle By Name(cluster=w121, "Steps"=w114, "Cycles"=w113, "Sweep type"=2, "Freq"=w116, "Start ampl"=w109, "Stop ampl"=w108, "Resolution"=u16 5) -> (w119:T1)
            }
            frame "wavefile" {
              w130 = T5 {"Level(U)"=0.0, "Wave Path"="", "ML axis"=1, "ML val level name"="", "Use ML Val level?"=FALSE, "wave info"="", "wave time"="", "Peak value4"=0.0, "RMS value4"=0.0, "wave channel"=0, "unit"=0, "Output Imp"=0.0, "Nominal Imp"=0.0, "V on DUT"=FALSE}  # wavefile
              n35 = Unflatten From String(type=T15 {"Level(U)"=0.0, "Wave Path"="", "ML axis"=1, "ML val level name"="", "Use ML Val level?"=FALSE, "wave info"="", "wave time"="", "Peak value4"=0.0, "RMS value4"=0.0} ("wavefile"), binary string=w148) -> (value=w147:T15)  [unwired: 1 in, 4 out]
              n36 = Unbundle By Name(w147) -> ("Level(U)"=w139:dbl, "Wave Path"=w138:string, "Use ML Val level?"=w137:bool, "ML axis"=w136:u8, "ML val level name"=w135:string)
              n37 = Bundle By Name(cluster=w130, "Level(U)"=w139, "Wave Path"=w138, "Use ML Val level?"=w137, "ML axis"=w136, "ML val level name"=w135, "wave channel"=0, "unit"=u16 0) -> (w133:T5)
              n38 = property on="wavefile" class="Clust (strict)"("Value"=w133) -> ()  [unwired: 2 in, 2 out]
              n39 = case shown="True" w137 {
                tunnel: w136 -> [_ w153]
                tunnel: w139 -> [w150 _]
                tunnel: [w150 w151] -> w140
                tunnel: w135 -> [_ w152]
                frame False {
                }
                frame True {
                  n40 = call "CRYGet Value from Curve Name.vi"("ML axis"=w153, "Level Name"=w152) -> ("Linear Value"=w151:dbl)  [unwired: 9 in]
                }
              }
              n41 = Bundle By Name(cluster=w145, "Level Out"=w140, "wav path"=w138, "Sweep type"=3, "Resolution"=u16 5, "Steps"=u32 1, "Tone type6"=u16 0) -> (w146:T1)
            }
            frame "dcconn" {
              w164 = T6 {"dc ctrl"=0, "dcmax I"=0, "dc polar"=0, "dc ctrl"=0, "Steps (#)"=19, "Time/step (s)"=0.05, "Start Ampl(U)"=1.0, "Stop Ampl(U)"=1.0, "Level(U)"=1.0, "Step Size"=1.0}  # dcconn
              n42 = Unflatten From String(type=T16 {"dc ctrl"=0, "dcmax I"=0, "dc polar"=0, "dc ctrl"=0, "Steps (#)"=19, "Time/step (s)"=0.05, "Start Ampl(U)"=1.0, "Stop Ampl(U)"=1.0, "Level(U)"=1.0, "Step Size"=1.0} ("dcconn"), binary string=w174) -> (value=w171:T16)  [unwired: 1 in, 4 out]
              n43 = Unbundle By Name(w171) -> ("dc ctrl"=w163:u16, "dcmax I"=w162:u16, "dc polar"=w161:u16, "dc ctrl"=w160:u16, "Steps (#)"=w159:i32, "Time/step (s)"=w158:dbl, "Start Ampl(U)"=w157:dbl, "Stop Ampl(U)"=w156:dbl, "Level(U)"=w155:dbl, "Step Size"=w154:dbl)
              n44 = Bundle By Name(cluster=w164, "dc ctrl"=w163, "dcmax I"=w162, "dc polar"=w161, "dc ctrl"=w160, "Steps (#)"=w159, "Time/step (s)"=w158, "Start Ampl(U)"=w157, "Stop Ampl(U)"=w156, "Level(U)"=w155, "Step Size"=w154) -> (w165:T6)
              n45 = Bundle By Name(cluster=w173, "Sweep type"=4, "Start ampl"=w157, "Stop ampl"=w156, "Sweep time"=w158, "Resolution"=u16 5, "Steps"=u32 1) -> (w172:T1)
              n46 = property on="dcconn" class="Clust (strict)"("Value"=w165) -> ()  [unwired: 2 in, 2 out]
            }
            frame "twotone" {
              w177 = T7 {"Steps (#)"=19, "Tone Type"=0, "Freq2(Hz)"=1000.0, "Time/step (s)"=0.0, "Cycles/step (#)"=12, "ML val level name"="", "Use ML Val level?"=FALSE, "Level(U) 2"=1.0, "Diff Freq(Hz)"=100.0, "ML axis 2"=1, "Diff/Ratio"=0, "Level(U)"=1.0, "Stop Freq(Hz)"=100.0, "Ratio Val"=0.8, "ML val level name 2"="", "Use ML Val level? 2"=FALSE, "ML axis"=1, "Start Freq(Hz)"=6300.0, "Step Resolution"=0, "Ratio"=0, "TabCtrl6"=enum."Master Tone", "unit 1"=0, "unit 2"=0, "Start Freq Name"="", "Stop Freq Name"="", "Start Freq Axis"=0, "Stop Freq Axis"=0, "Start Freq Flag"="", "Stop Freq Flag"=""}  # twotone
              w199 = u16 0 ("unit 1")
              n47 = Unflatten From String(type=T17 {"Steps (#)"=11, "Tone Type"=1, "Freq2(Hz)"=1000.0, "Time/step (s)"=1.0, "Cycles/step (#)"=10, "ML val level name"="unity cal(Read only) sens-out L", "Use ML Val level?"=TRUE, "Level(U) 2"=1.0, "Diff Freq(Hz)"=1.0, "ML axis 2"=0, "Diff/Ratio"=0, "Level(U)"=1.0, "Stop Freq(Hz)"=20.0, "Ratio Val"=0.0, "ML val level name 2"="unity cal(Read only) sens-out L", "Use ML Val level? 2"=TRUE, "ML axis"=0, "Start Freq(Hz)"=2.0, "Step Resolution"=0, "Ratio"=0, "TabCtrl6"=enum."Slave Tone"} ("twotone"), binary string=w208) -> (value=w205:T17)  [unwired: 1 in, 4 out]
              n48 = Unbundle By Name(w205) -> ("Level(U)"=w179:dbl, "Use ML Val level?"=w180:bool, "ML axis"=w181:u8, "ML val level name"=w182:string, "Start Freq(Hz)"=w183:dbl, "Stop Freq(Hz)"=w184:dbl, "Step Resolution"=w185:u16, "Steps (#)"=w186:i32, "Cycles/step (#)"=w187:u32, "Freq2(Hz)"=w188:dbl, "Level(U) 2"=w189:dbl, "Use ML Val level? 2"=w190:bool, "ML axis 2"=w191:u8, "ML val level name 2"=w192:string, "Diff Freq(Hz)"=w193:dbl, "Tone Type"=w194:u8, "Diff/Ratio"=w195:u8, "Ratio"=w196:u16, "Ratio Val"=w197:dbl, "Time/step (s)"=w198:dbl)
              n49 = Bundle By Name(cluster=w177, "Level(U)"=w179, "Use ML Val level?"=w180, "ML axis"=w181, "ML val level name"=w182, "Start Freq(Hz)"=w183, "Stop Freq(Hz)"=w184, "Step Resolution"=w185, "Steps (#)"=w186, "Cycles/step (#)"=w187, "Freq2(Hz)"=w188, "Level(U) 2"=w189, "Use ML Val level? 2"=w190, "ML axis"=w191, "ML val level name 2"=w192, "Diff Freq(Hz)"=w193, "Tone Type"=w194, "Diff/Ratio"=w195, "Ratio"=w196, "Ratio Val"=w197, "Time/step (s)"=w198, "unit 1"=w199, "unit 2"=w199) -> (w178:T7)
              n50 = case shown="True" w180 {
                tunnel: w181 -> [_ w217]
                tunnel: w179 -> [w214 _]
                tunnel: [w214 w215] -> w201
                tunnel: w182 -> [_ w216]
                frame False {
                }
                frame True {
                  n51 = call "CRYGet Value from Curve Name.vi"("ML axis"=w217, "Level Name"=w216) -> ("Linear Value"=w215:dbl)  [unwired: 9 in]
                }
              }
              n52 = case shown="True" w190 {
                tunnel: w191 -> [_ w213]
                tunnel: w189 -> [w210 _]
                tunnel: [w210 w211] -> w200
                tunnel: w192 -> [_ w212]
                frame False {
                }
                frame True {
                  n53 = call "CRYGet Value from Curve Name.vi"("ML axis"=w213, "Level Name"=w212) -> ("Linear Value"=w211:dbl)  [unwired: 9 in]
                }
              }
              n54 = To Double Precision Float(number=w188) -> (double precision float=w203:dbl)
              n55 = property on="twotone" class="Clust (strict)"("Value"=w178) -> ()  [unwired: 2 in, 2 out]
              n56 = Bundle By Name(cluster=w207, "Level Out"=w201, "Start Freq"=w183, "Stop Freq"=w184, "Resolution"=w185, "Steps"=w186, "Cycles"=w187, "Freq"=w203, "Start ampl"=w200, "Sweep type"=5, "Difference6"=w193, "Tone type6"=w194, "fix/ratio6"=w195, "Ratio6"=w196, "RatioFreq6"=w197, "Sweep time"=w198) -> (w206:T1)
            }
            frame "noise" {
              w219 = T9 {"Noise Type"=0, "Min Freq(Hz)"=20.0, "Max Freq(Hz)"=20000.0, "Level(U)"=1.0, "Duration(s)"=1.0, "ML val level name"="", "Use ML Val level?"=FALSE, "ML axis"=1, "unit"=0, "Start Freq Name"="", "Stop Freq Name"="", "Start Freq Axis"=0, "Stop Freq Axis"=0, "Start Freq Flag"="", "Stop Freq Flag"="", "Output Imp"=0.0, "Nominal Imp"=0.0, "V on DUT"=FALSE}  # noise
              n57 = Unflatten From String(type=T18 {"Noise Type"=0, "Min Freq(Hz)"=20.0, "Max Freq(Hz)"=20000.0, "Level(U)"=1.0, "Duration(s)"=1.0, "ML val level name"="", "Use ML Val level?"=FALSE, "ML axis"=1} ("noise"), binary string=w238) -> (value=w236:T18)  [unwired: 1 in, 4 out]
              n58 = Unbundle By Name(w236) -> ("Min Freq(Hz)"=w228:dbl, "Max Freq(Hz)"=w227:dbl, "Level(U)"=w226:dbl, "Duration(s)"=w225:dbl, "Noise Type"=w224:u8, "Use ML Val level?"=w223:bool, "ML axis"=w222:u8, "ML val level name"=w221:string)
              n59 = Bundle By Name(cluster=w219, "Min Freq(Hz)"=w228, "Max Freq(Hz)"=w227, "Level(U)"=w226, "Duration(s)"=w225, "Noise Type"=w224, "Use ML Val level?"=w223, "ML axis"=w222, "ML val level name"=w221, "unit"=u16 0) -> (w229:T9)
              n60 = property on="noise" class="Clust (strict)"("Value"=w229) -> ()  [unwired: 2 in, 2 out]
              n61 = case shown="True" w223 {
                tunnel: w222 -> [_ w243]
                tunnel: w226 -> [w240 _]
                tunnel: [w240 w241] -> w230
                tunnel: w221 -> [_ w242]
                frame False {
                }
                frame True {
                  n62 = call "CRYGet Value from Curve Name.vi"("ML axis"=w243, "Level Name"=w242) -> ("Linear Value"=w241:dbl)  [unwired: 9 in]
                }
              }
              n63 = Bundle By Name(cluster=w237, "Level Out"=w230, "Start Freq"=w228, "Stop Freq"=w227, "Sweep type"=6, "Sweep time"=w225, "Tone type6"=w224, "Resolution"=u16 5, "Steps"=u32 1) -> (w235:T1)
            }
            frame "mltitone" {
              w245 = T8 {"Level(U)"=0.0, "Min Freq(Hz)"=0.0, "Max Freq(Hz)"=0.0, "Duration(s)"=0.0, "Freq Rounding"=FALSE, "Rounding Val"=5.0, "Profile"=0, "ML axis 2"=0, "ML val level name"="", "Use ML Val level?"=FALSE, "ML axis"=0, "Step Resolution"=0, "unit"=0, "Start Freq Name"="Calibration sens-out Left", "Stop Freq Name"="Calibration sens-out Left", "Start Freq Axis"=0, "Stop Freq Axis"=0, "Start Freq Flag"="", "Stop Freq Flag"="", "Output Imp"=0.0, "Nominal Imp"=0.0, "V on DUT"=FALSE}  # mltitone
              n64 = Unflatten From String(type=T19 {"Level(U)"=0.0, "Min Freq(Hz)"=0.0, "Max Freq(Hz)"=0.0, "Duration(s)"=0.0, "Freq Rounding"=FALSE, "Rounding Val"=0.0, "Profile"=0, "ML axis 2"=0, "ML val level name"="", "Use ML Val level?"=FALSE, "ML axis"=0, "Step Resolution"=0} ("mltitone"), binary string=w266) -> (value=w265:T19)  [unwired: 1 in, 4 out]
              n65 = Unbundle By Name(w265) -> ("Level(U)"=w259:dbl, "Min Freq(Hz)"=w258:dbl, "Max Freq(Hz)"=w257:dbl, "Profile"=w256:i32, "Duration(s)"=w255:dbl, "Step Resolution"=w254:u16, "Use ML Val level?"=w253:bool, "ML axis"=w252:u8, "ML val level name"=w251:string)
              n66 = Bundle By Name(cluster=w245, "Level(U)"=w259, "Min Freq(Hz)"=w258, "Max Freq(Hz)"=w257, "Profile"=w256, "Duration(s)"=w255, "Step Resolution"=w254, "Use ML Val level?"=w253, "ML axis"=w252, "ML val level name"=w251, "unit"=u16 0, "Freq Rounding"=FALSE, "Rounding Val"=0.0, "ML axis 2"=u8 0) -> (w246:T8)
              n67 = property on="mltitone" class="Clust (strict)"("Value"=w246) -> ()  [unwired: 2 in, 2 out]
              n68 = case shown="True" w253 {
                tunnel: w252 -> [_ w271]
                tunnel: w259 -> [w268 _]
                tunnel: [w268 w269] -> w260
                tunnel: w251 -> [_ w270]
                frame False {
                }
                frame True {
                  n69 = call "CRYGet Value from Curve Name.vi"("ML axis"=w271, "Level Name"=w270) -> ("Linear Value"=w269:dbl)  [unwired: 9 in]
                }
              }
              n70 = Bundle By Name(cluster=w264, "Level Out"=w260, "Start Freq"=w258, "Stop Freq"=w257, "Steps"=w256, "Sweep time"=w255, "Resolution"=w254, "Sweep type"=7) -> (w263:T1)
            }
          }
        }
        frame 2 {
          n71 = case shown="\"flogsw\"" w274 {
            tunnel: w278 -> [_ w303 w329 w354 w377 w403 w437 w467 w495]
            tunnel: [errorcluster {"status"=TRUE, "code"=0, "source"=""} ("error in (no error)") w302 w328 w353 w378 w404 w438 w468 w496] -> w277
            tunnel: w276 -> [_ w302 w328 w353 w378 w404 w438 w468 w496]
            tunnel: w272 -> [w280 w298 w326 w351 w375 w402 w436 w466 w493]
            tunnel: [w280 w300 w324 w349 w376 w401 w435 w464 w492] -> w275
            tunnel: ["" "Frequency Stepped Sweep" "Frequency Log Sweep" "Log Amplitude Sweep" "WAV" "DC Connect" "Two Tone" "Noise" "Multitone"] -> w273
            frame Default {
            }
            frame "fstepsw" {
              w283 = T2 {"Level(U)"=0.7071067811865476, "Start Freq(Hz)"=20000.0, "Stop Freq(Hz)"=20.0, "ML val level name"="Calibration sens-out Left", "Use ML Val level?"=FALSE, "ML axis"=0, "Steps (#)"=31, "Cycles/step(#)"=20, "Time/step (s)"=0.01, "Step Resolution"=0, "unit"=0, "Start Freq Name"="Calibration sens-out Left", "Stop Freq Name"="Calibration sens-out Left", "Start Freq Axis"=0, "Stop Freq Axis"=0, "Start Freq Flag"="", "Stop Freq Flag"="", "Output Imp"=0.0, "Nominal Imp"=0.0, "V on DUT"=FALSE}  # fstepsw 4.0
              n72 = Unflatten From String(type=T12 {"Level(U)"=1.0, "Start Freq(Hz)"=6300.0, "Stop Freq(Hz)"=100.0, "ML val level name"="", "Use ML Val level?"=FALSE, "ML axis"=1, "Steps (#)"=19, "Cycles/step(#)"=8, "Time/step (s)"=0.01, "Step Resolution"=0} ("fstepsw"), binary string=w303) -> (value=w299:T12)  [unwired: 1 in, 4 out]
              n73 = Unbundle By Name(w299) -> ("Start Freq(Hz)"=w294:dbl, "Stop Freq(Hz)"=w293:dbl, "Steps (#)"=w292:i32, "Step Resolution"=w291:u16, "Cycles/step(#)"=w290:u32, "Time/step (s)"=w289:dbl, "Level(U)"=w288:dbl, "Use ML Val level?"=w287:bool, "ML axis"=w286:u8, "ML val level name"=w285:string)
              n74 = Bundle By Name(cluster=w283, "Start Freq(Hz)"=w294, "Stop Freq(Hz)"=w293, "Steps (#)"=w292, "Step Resolution"=w291, "Cycles/step(#)"=w290, "Time/step (s)"=w289, "Level(U)"=w288, "Use ML Val level?"=w287, "ML axis"=w286, "ML val level name"=w285, "unit"=u16 0) -> (w295:T2)
              n75 = property on="fstepsw" class="Clust (strict)"("Value"=w295) -> ()  [unwired: 2 in, 2 out]
              n76 = case shown="True" w287 {
                tunnel: w286 -> [_ w307]
                tunnel: w288 -> [w304 _]
                tunnel: [w304 w305] -> w296
                tunnel: w285 -> [_ w306]
                frame False {
                }
                frame True {
                  n77 = call "CRYGet Value from Curve Name.vi"("ML axis"=w307, "Level Name"=w306) -> ("Linear Value"=w305:dbl)  [unwired: 9 in]
                }
              }
              n78 = Bundle By Name(cluster=w298, "Start Freq"=w294, "Stop Freq"=w293, "Resolution"=w291, "Steps"=w292, "Cycles"=w290, "Sweep type"=0, "Sweep time"=w289, "Level Out"=w296) -> (w300:T1)
            }
            frame "flogsw" {
              w309 = T3 {"Level(U)"=1.0, "Start Freq(Hz)"=100.0, "Stop Freq(Hz)"=6300.0, "Sweep Rate(s/dec)"=1.0, "Use ML Val level?"=FALSE, "ML val level name"="", "ML axis"=1, "TSR params"={"FSamp"=0.0, "FStart"=0.0, "FStop"=0.0, "NOffset"=0.0, "MStop"=0.0, "MStart"=0.0, "NHarm"=0.0, "Tsamp"=0.0, "Amplit"=0.0}, "unit"=0, "Start Freq Name"="Calibration sens-out Left", "Stop Freq Name"="Calibration sens-out Left", "Start Freq Axis"=0, "Stop Freq Axis"=0, "Start Freq Flag"="", "Stop Freq Flag"="", "Output Imp"=0.0, "Nominal Imp"=0.0, "V on DUT"=FALSE}  # flogsw
              n79 = Unflatten From String(type=T13 {"Level(U)"=1.0, "Start Freq(Hz)"=100.0, "Stop Freq(Hz)"=6300.0, "Sweep Rate(s/dec)"=1.0, "Use ML Val level?"=FALSE, "ML val level name"="", "ML axis"=1, "TSR params"={"FSamp"=0.0, "FStart"=0.0, "FStop"=0.0, "NOffset"=0.0, "MStop"=0.0, "MStart"=0.0, "NHarm"=0.0, "Tsamp"=0.0, "Amplit"=0.0}} ("flogsw"), binary string=w329) -> (value=w327:T13)  [unwired: 1 in, 4 out]
              n80 = Unbundle By Name(w327) -> ("Level(U)"=w318:dbl, "Start Freq(Hz)"=w317:dbl, "Stop Freq(Hz)"=w316:dbl, "Sweep Rate(s/dec)"=w315:dbl, "Use ML Val level?"=w314:bool, "ML axis"=w313:u8, "ML val level name"=w312:string, "TSR params"=w311:T29)
              n81 = Bundle By Name(cluster=w309, "Level(U)"=w318, "Start Freq(Hz)"=w317, "Stop Freq(Hz)"=w316, "Sweep Rate(s/dec)"=w315, "Use ML Val level?"=w314, "ML axis"=w313, "ML val level name"=w312, "TSR params"=w311, "unit"=u16 0) -> (w319:T3)
              n82 = property on="flogsw" class="Clust (strict)"("Value"=w319) -> ()  [unwired: 2 in, 2 out]
              n83 = case shown="True" w314 {
                tunnel: w313 -> [_ w333]
                tunnel: w318 -> [w330 _]
                tunnel: [w330 w331] -> w320
                tunnel: w312 -> [_ w332]
                frame False {
                }
                frame True {
                  n84 = call "CRYGet Value from Curve Name.vi"("ML axis"=w333, "Level Name"=w332) -> ("Linear Value"=w331:dbl)  [unwired: 9 in]
                }
              }
              n85 = Bundle By Name(cluster=w326, "Level Out"=w320, "Start Freq"=w317, "Stop Freq"=w316, "Sweep type"=1, "Sweep time"=w315, "Resolution"=u16 5, "Steps"=u32 1) -> (w324:T1)
            }
            frame "ampsw" {
              w335 = T4 {"Freq(Hz)"=1000.0, "Steps (#)"=19, "Cycles(#)"=12, "Use ML Val freq?"=FALSE, "ML val freq name"="", "ML axis"=1, "Start Ampl(U)"=0.5, "Stop Ampl(U)"=1.0, "unit"=0}  # ampsw
              n86 = Unflatten From String(type=T14 {"Freq(Hz)"=1000.0, "Steps (#)"=19, "Cycles(#)"=12, "Use ML Val freq?"=FALSE, "ML val freq name"="", "ML axis"=1, "Start Ampl(U)"=0.5, "Stop Ampl(U)"=1.0} ("ampsw"), binary string=w354) -> (value=w352:T14)  [unwired: 1 in, 4 out]
              n87 = Unbundle By Name(w352) -> ("Freq(Hz)"=w344:dbl, "Steps (#)"=w343:i32, "Cycles(#)"=w342:u32, "Use ML Val freq?"=w341:bool, "ML axis"=w340:u8, "ML val freq name"=w339:string, "Start Ampl(U)"=w338:dbl, "Stop Ampl(U)"=w337:dbl)
              n88 = Bundle By Name(cluster=w335, "Freq(Hz)"=w344, "Steps (#)"=w343, "Cycles(#)"=w342, "Use ML Val freq?"=w341, "ML axis"=w340, "ML val freq name"=w339, "Start Ampl(U)"=w338, "Stop Ampl(U)"=w337, "unit"=u16 0) -> (w345:T4)
              n89 = property on="ampsw" class="Clust (strict)"("Value"=w345) -> ()  [unwired: 2 in, 2 out]
              n90 = case shown="True" w341 {
                tunnel: w340 -> [_ w358]
                tunnel: w344 -> [w355 _]
                tunnel: [w355 w356] -> w346
                tunnel: w339 -> [_ w357]
                frame False {
                }
                frame True {
                  n91 = call "CRYGet Value from Curve Name.vi"("ML axis"=w358, "Level Name"=w357) -> ("Linear Value"=w356:dbl)  [unwired: 9 in]
                }
              }
              n92 = Bundle By Name(cluster=w351, "Steps"=w343, "Cycles"=w342, "Sweep type"=2, "Freq"=w346, "Start ampl"=w338, "Stop ampl"=w337, "Resolution"=u16 5) -> (w349:T1)
            }
            frame "wavefile" {
              w360 = T5 {"Level(U)"=0.0, "Wave Path"="", "ML axis"=1, "ML val level name"="", "Use ML Val level?"=FALSE, "wave info"="", "wave time"="", "Peak value4"=0.0, "RMS value4"=0.0, "wave channel"=0, "unit"=0, "Output Imp"=0.0, "Nominal Imp"=0.0, "V on DUT"=FALSE}  # wavefile
              n93 = Unflatten From String(type=T20 {"Level(U)"=0.0, "Wave Path"="", "ML axis"=1, "ML val level name"="", "Use ML Val level?"=FALSE, "wave info"="", "wave time"="", "Peak value4"=0.0, "RMS value4"=0.0, "wave channel"=19} ("wavefile"), binary string=w377) -> (value=w369:T20)  [unwired: 1 in, 4 out]
              n94 = Unbundle By Name(w369) -> ("Level(U)"=w366:dbl, "Wave Path"=w365:string, "Use ML Val level?"=w364:bool, "ML axis"=w363:u8, "ML val level name"=w362:string, "wave channel"=w361:u16)
              n95 = Bundle By Name(cluster=w360, "Level(U)"=w366, "Wave Path"=w365, "Use ML Val level?"=w364, "ML axis"=w363, "ML val level name"=w362, "wave channel"=w361, "unit"=u16 0) -> (w367:T5)
              n96 = property on="wavefile" class="Clust (strict)"("Value"=w367) -> ()  [unwired: 2 in, 2 out]
              n97 = case shown="True" w364 {
                tunnel: w363 -> [_ w382]
                tunnel: w366 -> [w379 _]
                tunnel: [w379 w380] -> w370
                tunnel: w362 -> [_ w381]
                frame False {
                }
                frame True {
                  n98 = call "CRYGet Value from Curve Name.vi"("ML axis"=w382, "Level Name"=w381) -> ("Linear Value"=w380:dbl)  [unwired: 9 in]
                }
              }
              n99 = Bundle By Name(cluster=w375, "Level Out"=w370, "wav path"=w365, "Sweep type"=3, "Resolution"=u16 5, "Steps"=u32 1, "Tone type6"=w361) -> (w376:T1)
            }
            frame "dcconn" {
              w394 = T6 {"dc ctrl"=0, "dcmax I"=0, "dc polar"=0, "dc ctrl"=0, "Steps (#)"=19, "Time/step (s)"=0.05, "Start Ampl(U)"=1.0, "Stop Ampl(U)"=1.0, "Level(U)"=1.0, "Step Size"=1.0}  # dcconn
              n100 = Unflatten From String(type=T16 {"dc ctrl"=0, "dcmax I"=0, "dc polar"=0, "dc ctrl"=0, "Steps (#)"=19, "Time/step (s)"=0.05, "Start Ampl(U)"=1.0, "Stop Ampl(U)"=1.0, "Level(U)"=1.0, "Step Size"=1.0} ("dcconn"), binary string=w403) -> (value=w400:T16)  [unwired: 1 in, 4 out]
              n101 = Unbundle By Name(w400) -> ("dc ctrl"=w392:u16, "dcmax I"=w391:u16, "dc polar"=w390:u16, "dc ctrl"=w389:u16, "Steps (#)"=w388:i32, "Time/step (s)"=w387:dbl, "Start Ampl(U)"=w386:dbl, "Stop Ampl(U)"=w385:dbl, "Level(U)"=w384:dbl, "Step Size"=w383:dbl)
              n102 = Bundle By Name(cluster=w394, "dc ctrl"=w392, "dcmax I"=w391, "dc polar"=w390, "dc ctrl"=w389, "Steps (#)"=w388, "Time/step (s)"=w387, "Start Ampl(U)"=w386, "Stop Ampl(U)"=w385, "Level(U)"=w384, "Step Size"=w383) -> (w395:T6)
              n103 = Bundle By Name(cluster=w402, "Sweep type"=4, "Start ampl"=w386, "Stop ampl"=w385, "Sweep time"=w387, "Resolution"=u16 5, "Steps"=u32 1) -> (w401:T1)
              n104 = property on="dcconn" class="Clust (strict)"("Value"=w395) -> ()  [unwired: 2 in, 2 out]
            }
            frame "twotone" {
              w407 = T7 {"Steps (#)"=19, "Tone Type"=0, "Freq2(Hz)"=1000.0, "Time/step (s)"=0.0, "Cycles/step (#)"=12, "ML val level name"="", "Use ML Val level?"=FALSE, "Level(U) 2"=1.0, "Diff Freq(Hz)"=100.0, "ML axis 2"=1, "Diff/Ratio"=0, "Level(U)"=1.0, "Stop Freq(Hz)"=100.0, "Ratio Val"=0.8, "ML val level name 2"="", "Use ML Val level? 2"=FALSE, "ML axis"=1, "Start Freq(Hz)"=6300.0, "Step Resolution"=0, "Ratio"=0, "TabCtrl6"=enum."Master Tone", "unit 1"=0, "unit 2"=0, "Start Freq Name"="", "Stop Freq Name"="", "Start Freq Axis"=0, "Stop Freq Axis"=0, "Start Freq Flag"="", "Stop Freq Flag"=""}  # twotone
              w428 = u16 0 ("unit 1")
              n105 = Unflatten From String(type=T17 {"Steps (#)"=11, "Tone Type"=1, "Freq2(Hz)"=1000.0, "Time/step (s)"=1.0, "Cycles/step (#)"=10, "ML val level name"="unity cal(Read only) sens-out L", "Use ML Val level?"=TRUE, "Level(U) 2"=1.0, "Diff Freq(Hz)"=1.0, "ML axis 2"=0, "Diff/Ratio"=0, "Level(U)"=1.0, "Stop Freq(Hz)"=20.0, "Ratio Val"=0.0, "ML val level name 2"="unity cal(Read only) sens-out L", "Use ML Val level? 2"=TRUE, "ML axis"=0, "Start Freq(Hz)"=2.0, "Step Resolution"=0, "Ratio"=0, "TabCtrl6"=enum."Slave Tone"} ("twotone"), binary string=w437) -> (value=w405:T17)  [unwired: 1 in, 4 out]
              n106 = Unbundle By Name(w405) -> ("Level(U)"=w427:dbl, "Use ML Val level?"=w426:bool, "ML axis"=w425:u8, "ML val level name"=w424:string, "Start Freq(Hz)"=w423:dbl, "Stop Freq(Hz)"=w422:dbl, "Step Resolution"=w421:u16, "Steps (#)"=w420:i32, "Cycles/step (#)"=w419:u32, "Freq2(Hz)"=w418:dbl, "Level(U) 2"=w417:dbl, "Use ML Val level? 2"=w416:bool, "ML axis 2"=w415:u8, "ML val level name 2"=w414:string, "Diff Freq(Hz)"=w413:dbl, "Tone Type"=w412:u8, "Diff/Ratio"=w411:u8, "Ratio"=w410:u16, "Ratio Val"=w409:dbl, "Time/step (s)"=w408:dbl)
              n107 = Bundle By Name(cluster=w407, "Level(U)"=w427, "Use ML Val level?"=w426, "ML axis"=w425, "ML val level name"=w424, "Start Freq(Hz)"=w423, "Stop Freq(Hz)"=w422, "Step Resolution"=w421, "Steps (#)"=w420, "Cycles/step (#)"=w419, "Freq2(Hz)"=w418, "Level(U) 2"=w417, "Use ML Val level? 2"=w416, "ML axis"=w415, "ML val level name 2"=w414, "Diff Freq(Hz)"=w413, "Tone Type"=w412, "Diff/Ratio"=w411, "Ratio"=w410, "Ratio Val"=w409, "Time/step (s)"=w408, "unit 1"=w428, "unit 2"=w428) -> (w429:T7)
              n108 = property on="twotone" class="Clust (strict)"("Value"=w429) -> ()  [unwired: 2 in, 2 out]
              n109 = case shown="True" w426 {
                tunnel: w425 -> [_ w446]
                tunnel: w427 -> [w443 _]
                tunnel: [w443 w444] -> w431
                tunnel: w424 -> [_ w445]
                frame False {
                }
                frame True {
                  n110 = call "CRYGet Value from Curve Name.vi"("ML axis"=w446, "Level Name"=w445) -> ("Linear Value"=w444:dbl)  [unwired: 9 in]
                }
              }
              n111 = case shown="True" w416 {
                tunnel: w415 -> [_ w442]
                tunnel: w417 -> [w439 _]
                tunnel: [w439 w440] -> w430
                tunnel: w414 -> [_ w441]
                frame False {
                }
                frame True {
                  n112 = call "CRYGet Value from Curve Name.vi"("ML axis"=w442, "Level Name"=w441) -> ("Linear Value"=w440:dbl)  [unwired: 9 in]
                }
              }
              n113 = To Double Precision Float(number=w418) -> (double precision float=w433:dbl)
              n114 = Bundle By Name(cluster=w436, "Level Out"=w431, "Start Freq"=w423, "Stop Freq"=w422, "Resolution"=w421, "Steps"=w420, "Cycles"=w419, "Freq"=w433, "Start ampl"=w430, "Sweep type"=5, "Difference6"=w413, "Tone type6"=w412, "fix/ratio6"=w411, "Ratio6"=w410, "RatioFreq6"=w409, "Sweep time"=w408) -> (w435:T1)
            }
            frame "noise" {
              w448 = T9 {"Noise Type"=0, "Min Freq(Hz)"=20.0, "Max Freq(Hz)"=20000.0, "Level(U)"=1.0, "Duration(s)"=1.0, "ML val level name"="", "Use ML Val level?"=FALSE, "ML axis"=1, "unit"=0, "Start Freq Name"="", "Stop Freq Name"="", "Start Freq Axis"=0, "Stop Freq Axis"=0, "Start Freq Flag"="", "Stop Freq Flag"="", "Output Imp"=0.0, "Nominal Imp"=0.0, "V on DUT"=FALSE}  # noise
              n115 = Unflatten From String(type=T18 {"Noise Type"=0, "Min Freq(Hz)"=20.0, "Max Freq(Hz)"=20000.0, "Level(U)"=1.0, "Duration(s)"=1.0, "ML val level name"="", "Use ML Val level?"=FALSE, "ML axis"=1} ("noise"), binary string=w467) -> (value=w465:T18)  [unwired: 1 in, 4 out]
              n116 = Unbundle By Name(w465) -> ("Min Freq(Hz)"=w458:dbl, "Max Freq(Hz)"=w457:dbl, "Level(U)"=w456:dbl, "Duration(s)"=w455:dbl, "Noise Type"=w454:u8, "Use ML Val level?"=w453:bool, "ML axis"=w452:u8, "ML val level name"=w451:string)
              n117 = Bundle By Name(cluster=w448, "Min Freq(Hz)"=w458, "Max Freq(Hz)"=w457, "Level(U)"=w456, "Duration(s)"=w455, "Noise Type"=w454, "Use ML Val level?"=w453, "ML axis"=w452, "ML val level name"=w451, "unit"=u16 0) -> (w449:T9)
              n118 = property on="noise" class="Clust (strict)"("Value"=w449) -> ()  [unwired: 2 in, 2 out]
              n119 = case shown="True" w453 {
                tunnel: w452 -> [_ w472]
                tunnel: w456 -> [w469 _]
                tunnel: [w469 w470] -> w459
                tunnel: w451 -> [_ w471]
                frame False {
                }
                frame True {
                  n120 = call "CRYGet Value from Curve Name.vi"("ML axis"=w472, "Level Name"=w471) -> ("Linear Value"=w470:dbl)  [unwired: 9 in]
                }
              }
              n121 = Bundle By Name(cluster=w466, "Level Out"=w459, "Start Freq"=w458, "Stop Freq"=w457, "Sweep type"=6, "Sweep time"=w455, "Tone type6"=w454, "Resolution"=u16 5, "Steps"=u32 1) -> (w464:T1)
            }
            frame "mltitone" {
              w474 = T8 {"Level(U)"=0.0, "Min Freq(Hz)"=0.0, "Max Freq(Hz)"=0.0, "Duration(s)"=0.0, "Freq Rounding"=FALSE, "Rounding Val"=5.0, "Profile"=0, "ML axis 2"=0, "ML val level name"="", "Use ML Val level?"=FALSE, "ML axis"=0, "Step Resolution"=0, "unit"=0, "Start Freq Name"="Calibration sens-out Left", "Stop Freq Name"="Calibration sens-out Left", "Start Freq Axis"=0, "Stop Freq Axis"=0, "Start Freq Flag"="", "Stop Freq Flag"="", "Output Imp"=0.0, "Nominal Imp"=0.0, "V on DUT"=FALSE}  # mltitone
              n122 = Unflatten From String(type=T19 {"Level(U)"=0.0, "Min Freq(Hz)"=0.0, "Max Freq(Hz)"=0.0, "Duration(s)"=0.0, "Freq Rounding"=FALSE, "Rounding Val"=0.0, "Profile"=0, "ML axis 2"=0, "ML val level name"="", "Use ML Val level?"=FALSE, "ML axis"=0, "Step Resolution"=0} ("mltitone"), binary string=w495) -> (value=w494:T19)  [unwired: 1 in, 4 out]
              n123 = Unbundle By Name(w494) -> ("Level(U)"=w483:dbl, "Min Freq(Hz)"=w482:dbl, "Max Freq(Hz)"=w481:dbl, "Profile"=w480:i32, "Duration(s)"=w479:dbl, "Step Resolution"=w478:u16, "Use ML Val level?"=w477:bool, "ML axis"=w476:u8, "ML val level name"=w475:string)
              n124 = Bundle By Name(cluster=w474, "Level(U)"=w483, "Min Freq(Hz)"=w482, "Max Freq(Hz)"=w481, "Profile"=w480, "Duration(s)"=w479, "Step Resolution"=w478, "Use ML Val level?"=w477, "ML axis"=w476, "ML val level name"=w475, "unit"=u16 0, "Freq Rounding"=FALSE, "Rounding Val"=0.0, "ML axis 2"=u8 0) -> (w484:T8)
              n125 = property on="mltitone" class="Clust (strict)"("Value"=w484) -> ()  [unwired: 2 in, 2 out]
              n126 = case shown="True" w477 {
                tunnel: w476 -> [_ w500]
                tunnel: w483 -> [w497 _]
                tunnel: [w497 w498] -> w489
                tunnel: w475 -> [_ w499]
                frame False {
                }
                frame True {
                  n127 = call "CRYGet Value from Curve Name.vi"("ML axis"=w500, "Level Name"=w499) -> ("Linear Value"=w498:dbl)  [unwired: 9 in]
                }
              }
              n128 = Bundle By Name(cluster=w493, "Level Out"=w489, "Start Freq"=w482, "Stop Freq"=w481, "Steps"=w480, "Sweep time"=w479, "Resolution"=w478, "Sweep type"=7) -> (w492:T1)
            }
          }
        }
        frame 3 {
          n129 = case shown="\"fstepsw\"" w503 {
            tunnel: w507 -> [_ w532 w558 w583 w606 w632 w667 w697 w725]
            tunnel: [errorcluster {"status"=TRUE, "code"=0, "source"=""} ("error in (no error)") w531 w557 w582 w607 w633 w668 w698 w726] -> w506
            tunnel: w505 -> [_ w531 w557 w582 w607 w633 w668 w698 w726]
            tunnel: w501 -> [w509 w527 w555 w580 w604 w631 w666 w696 w723]
            tunnel: [w509 w529 w553 w578 w605 w630 w665 w694 w722] -> w504
            tunnel: ["" "Frequency Stepped Sweep" "Frequency Log Sweep" "Log Amplitude Sweep" "WAV" "DC Connect" "Two Tone" "Noise" "Multitone"] -> w502
            frame Default {
            }
            frame "fstepsw" {
              w513 = T2 {"Level(U)"=0.7071067811865476, "Start Freq(Hz)"=20000.0, "Stop Freq(Hz)"=20.0, "ML val level name"="Calibration sens-out Left", "Use ML Val level?"=FALSE, "ML axis"=0, "Steps (#)"=31, "Cycles/step(#)"=20, "Time/step (s)"=0.01, "Step Resolution"=0, "unit"=0, "Start Freq Name"="Calibration sens-out Left", "Stop Freq Name"="Calibration sens-out Left", "Start Freq Axis"=0, "Stop Freq Axis"=0, "Start Freq Flag"="", "Stop Freq Flag"="", "Output Imp"=0.0, "Nominal Imp"=0.0, "V on DUT"=FALSE}  # fstepsw 4.0
              n130 = Unflatten From String(type=T21 {"Level(U)"=0.0, "Start Freq(Hz)"=0.0, "Stop Freq(Hz)"=0.0, "ML val level name"="", "Use ML Val level?"=FALSE, "ML axis"=0, "Steps (#)"=0, "Cycles/step(#)"=0, "Time/step (s)"=0.0, "Step Resolution"=0, "unit"=0} ("Value"), binary string=w532) -> (value=w528:T21)  [unwired: 1 in, 4 out]
              n131 = Unbundle By Name(w528) -> ("Start Freq(Hz)"=w523:dbl, "Stop Freq(Hz)"=w522:dbl, "Steps (#)"=w521:i32, "Step Resolution"=w520:u16, "Cycles/step(#)"=w519:u32, "Time/step (s)"=w518:dbl, "Level(U)"=w517:dbl, "Use ML Val level?"=w516:bool, "ML axis"=w515:u8, "ML val level name"=w514:string, "unit"=w511:u16)
              n132 = Bundle By Name(cluster=w513, "Start Freq(Hz)"=w523, "Stop Freq(Hz)"=w522, "Steps (#)"=w521, "Step Resolution"=w520, "Cycles/step(#)"=w519, "Time/step (s)"=w518, "Level(U)"=w517, "Use ML Val level?"=w516, "ML axis"=w515, "ML val level name"=w514, "unit"=w511) -> (w524:T2)
              n133 = property on="fstepsw" class="Clust (strict)"("Value"=w524) -> ()  [unwired: 2 in, 2 out]
              n134 = case shown="True" w516 {
                tunnel: w515 -> [_ w536]
                tunnel: w517 -> [w533 _]
                tunnel: [w533 w534] -> w525
                tunnel: w514 -> [_ w535]
                frame False {
                }
                frame True {
                  n135 = call "CRYGet Value from Curve Name.vi"("ML axis"=w536, "Level Name"=w535) -> ("Linear Value"=w534:dbl)  [unwired: 9 in]
                }
              }
              n136 = Bundle By Name(cluster=w527, "Start Freq"=w523, "Stop Freq"=w522, "Resolution"=w520, "Steps"=w521, "Cycles"=w519, "Sweep type"=0, "Sweep time"=w518, "Level Out"=w525) -> (w529:T1)
            }
            frame "flogsw" {
              w539 = T3 {"Level(U)"=1.0, "Start Freq(Hz)"=100.0, "Stop Freq(Hz)"=6300.0, "Sweep Rate(s/dec)"=1.0, "Use ML Val level?"=FALSE, "ML val level name"="", "ML axis"=1, "TSR params"={"FSamp"=0.0, "FStart"=0.0, "FStop"=0.0, "NOffset"=0.0, "MStop"=0.0, "MStart"=0.0, "NHarm"=0.0, "Tsamp"=0.0, "Amplit"=0.0}, "unit"=0, "Start Freq Name"="Calibration sens-out Left", "Stop Freq Name"="Calibration sens-out Left", "Start Freq Axis"=0, "Stop Freq Axis"=0, "Start Freq Flag"="", "Stop Freq Flag"="", "Output Imp"=0.0, "Nominal Imp"=0.0, "V on DUT"=FALSE}  # flogsw
              n137 = Unflatten From String(type=T22 {"Level(U)"=0.0, "Start Freq(Hz)"=0.0, "Stop Freq(Hz)"=0.0, "Sweep Rate(s/dec)"=0.0, "Use ML Val level?"=FALSE, "ML val level name"="", "ML axis"=0, "TSR params"={"FSamp"=0.0, "FStart"=0.0, "FStop"=0.0, "NOffset"=0.0, "MStop"=0.0, "MStart"=0.0, "NHarm"=0.0, "Tsamp"=0.0, "Amplit"=0.0}, "unit"=0} ("Value"), binary string=w558) -> (value=w556:T22)  [unwired: 1 in, 4 out]
              n138 = Unbundle By Name(w556) -> ("Level(U)"=w547:dbl, "Start Freq(Hz)"=w546:dbl, "Stop Freq(Hz)"=w545:dbl, "Sweep Rate(s/dec)"=w544:dbl, "Use ML Val level?"=w543:bool, "ML axis"=w542:u8, "ML val level name"=w541:string, "TSR params"=w540:T29, "unit"=w537:u16)
              n139 = Bundle By Name(cluster=w539, "Level(U)"=w547, "Start Freq(Hz)"=w546, "Stop Freq(Hz)"=w545, "Sweep Rate(s/dec)"=w544, "Use ML Val level?"=w543, "ML axis"=w542, "ML val level name"=w541, "TSR params"=w540, "unit"=w537) -> (w548:T3)
              n140 = property on="flogsw" class="Clust (strict)"("Value"=w548) -> ()  [unwired: 2 in, 2 out]
              n141 = case shown="True" w543 {
                tunnel: w542 -> [_ w562]
                tunnel: w547 -> [w559 _]
                tunnel: [w559 w560] -> w549
                tunnel: w541 -> [_ w561]
                frame False {
                }
                frame True {
                  n142 = call "CRYGet Value from Curve Name.vi"("ML axis"=w562, "Level Name"=w561) -> ("Linear Value"=w560:dbl)  [unwired: 9 in]
                }
              }
              n143 = Bundle By Name(cluster=w555, "Level Out"=w549, "Start Freq"=w546, "Stop Freq"=w545, "Sweep type"=1, "Sweep time"=w544, "Resolution"=u16 5, "Steps"=u32 1) -> (w553:T1)
            }
            frame "ampsw" {
              w565 = T4 {"Freq(Hz)"=1000.0, "Steps (#)"=19, "Cycles(#)"=12, "Use ML Val freq?"=FALSE, "ML val freq name"="", "ML axis"=1, "Start Ampl(U)"=0.5, "Stop Ampl(U)"=1.0, "unit"=0}  # ampsw
              n144 = Unflatten From String(type=T23 {"Freq(Hz)"=0.0, "Steps (#)"=0, "Cycles(#)"=0, "Use ML Val freq?"=FALSE, "ML val freq name"="", "ML axis"=0, "Start Ampl(U)"=0.0, "Stop Ampl(U)"=0.0, "unit"=0} ("Value"), binary string=w583) -> (value=w581:T23)  [unwired: 1 in, 4 out]
              n145 = Unbundle By Name(w581) -> ("Freq(Hz)"=w573:dbl, "Steps (#)"=w572:i32, "Cycles(#)"=w571:u32, "Use ML Val freq?"=w570:bool, "ML axis"=w569:u8, "ML val freq name"=w568:string, "Start Ampl(U)"=w567:dbl, "Stop Ampl(U)"=w566:dbl, "unit"=w563:u16)
              n146 = Bundle By Name(cluster=w565, "Freq(Hz)"=w573, "Steps (#)"=w572, "Cycles(#)"=w571, "Use ML Val freq?"=w570, "ML axis"=w569, "ML val freq name"=w568, "Start Ampl(U)"=w567, "Stop Ampl(U)"=w566, "unit"=w563) -> (w574:T4)
              n147 = property on="ampsw" class="Clust (strict)"("Value"=w574) -> ()  [unwired: 2 in, 2 out]
              n148 = case shown="True" w570 {
                tunnel: w569 -> [_ w587]
                tunnel: w573 -> [w584 _]
                tunnel: [w584 w585] -> w575
                tunnel: w568 -> [_ w586]
                frame False {
                }
                frame True {
                  n149 = call "CRYGet Value from Curve Name.vi"("ML axis"=w587, "Level Name"=w586) -> ("Linear Value"=w585:dbl)  [unwired: 9 in]
                }
              }
              n150 = Bundle By Name(cluster=w580, "Steps"=w572, "Cycles"=w571, "Sweep type"=2, "Freq"=w575, "Start ampl"=w567, "Stop ampl"=w566, "Resolution"=u16 5) -> (w578:T1)
            }
            frame "wavefile" {
              w590 = T5 {"Level(U)"=0.0, "Wave Path"="", "ML axis"=1, "ML val level name"="", "Use ML Val level?"=FALSE, "wave info"="", "wave time"="", "Peak value4"=0.0, "RMS value4"=0.0, "wave channel"=0, "unit"=0, "Output Imp"=0.0, "Nominal Imp"=0.0, "V on DUT"=FALSE}  # wavefile
              n151 = Unflatten From String(type=T24 {"Level(U)"=0.0, "Wave Path"="", "ML axis"=0, "ML val level name"="", "Use ML Val level?"=FALSE, "wave info"="", "wave time"="", "Peak value4"=0.0, "RMS value4"=0.0, "wave channel"=0, "unit"=0} ("Value"), binary string=w606) -> (value=w598:T24)  [unwired: 1 in, 4 out]
              n152 = Unbundle By Name(w598) -> ("Level(U)"=w596:dbl, "Wave Path"=w595:string, "Use ML Val level?"=w594:bool, "ML axis"=w593:u8, "ML val level name"=w592:string, "wave channel"=w591:u16, "unit"=w588:u16)
              n153 = Bundle By Name(cluster=w590, "Level(U)"=w596, "Wave Path"=w595, "Use ML Val level?"=w594, "ML axis"=w593, "ML val level name"=w592, "wave channel"=w591, "unit"=w588) -> (w597:T5)
              n154 = property on="wavefile" class="Clust (strict)"("Value"=w597) -> ()  [unwired: 2 in, 2 out]
              n155 = case shown="True" w594 {
                tunnel: w593 -> [_ w611]
                tunnel: w596 -> [w608 _]
                tunnel: [w608 w609] -> w599
                tunnel: w592 -> [_ w610]
                frame False {
                }
                frame True {
                  n156 = call "CRYGet Value from Curve Name.vi"("ML axis"=w611, "Level Name"=w610) -> ("Linear Value"=w609:dbl)  [unwired: 9 in]
                }
              }
              n157 = Bundle By Name(cluster=w604, "Level Out"=w599, "wav path"=w595, "Sweep type"=3, "Resolution"=u16 5, "Steps"=u32 1, "Tone type6"=w591) -> (w605:T1)
            }
            frame "dcconn" {
              w623 = T6 {"dc ctrl"=0, "dcmax I"=0, "dc polar"=0, "dc ctrl"=0, "Steps (#)"=19, "Time/step (s)"=0.05, "Start Ampl(U)"=1.0, "Stop Ampl(U)"=1.0, "Level(U)"=1.0, "Step Size"=1.0}  # dcconn
              n158 = Unflatten From String(type=T16 {"dc ctrl"=0, "dcmax I"=0, "dc polar"=0, "dc ctrl"=0, "Steps (#)"=0, "Time/step (s)"=0.0, "Start Ampl(U)"=0.0, "Stop Ampl(U)"=0.0, "Level(U)"=0.0, "Step Size"=0.0} ("Value"), binary string=w632) -> (value=w629:T16)  [unwired: 1 in, 4 out]
              n159 = Unbundle By Name(w629) -> ("dc ctrl"=w621:u16, "dcmax I"=w620:u16, "dc polar"=w619:u16, "dc ctrl"=w618:u16, "Steps (#)"=w617:i32, "Time/step (s)"=w616:dbl, "Start Ampl(U)"=w615:dbl, "Stop Ampl(U)"=w614:dbl, "Level(U)"=w613:dbl, "Step Size"=w612:dbl)
              n160 = Bundle By Name(cluster=w623, "dc ctrl"=w621, "dcmax I"=w620, "dc polar"=w619, "dc ctrl"=w618, "Steps (#)"=w617, "Time/step (s)"=w616, "Start Ampl(U)"=w615, "Stop Ampl(U)"=w614, "Level(U)"=w613, "Step Size"=w612) -> (w622:T6)
              n161 = Bundle By Name(cluster=w631, "Sweep type"=4, "Start ampl"=w615, "Stop ampl"=w614, "Sweep time"=w616, "Resolution"=u16 5, "Steps"=u32 1) -> (w630:T1)
              n162 = property on="dcconn" class="Clust (strict)"("Value"=w622) -> ()  [unwired: 2 in, 2 out]
            }
            frame "twotone" {
              w637 = T7 {"Steps (#)"=19, "Tone Type"=0, "Freq2(Hz)"=1000.0, "Time/step (s)"=0.0, "Cycles/step (#)"=12, "ML val level name"="", "Use ML Val level?"=FALSE, "Level(U) 2"=1.0, "Diff Freq(Hz)"=100.0, "ML axis 2"=1, "Diff/Ratio"=0, "Level(U)"=1.0, "Stop Freq(Hz)"=100.0, "Ratio Val"=0.8, "ML val level name 2"="", "Use ML Val level? 2"=FALSE, "ML axis"=1, "Start Freq(Hz)"=6300.0, "Step Resolution"=0, "Ratio"=0, "TabCtrl6"=enum."Master Tone", "unit 1"=0, "unit 2"=0, "Start Freq Name"="", "Stop Freq Name"="", "Start Freq Axis"=0, "Stop Freq Axis"=0, "Start Freq Flag"="", "Stop Freq Flag"=""}  # twotone
              n163 = Unflatten From String(type=T25 {"Steps (#)"=0, "Tone Type"=0, "Freq2(Hz)"=0.0, "Time/step (s)"=0.0, "Cycles/step (#)"=0, "ML val level name"="", "Use ML Val level?"=FALSE, "Level(U) 2"=0.0, "Diff Freq(Hz)"=0.0, "ML axis 2"=0, "Diff/Ratio"=0, "Level(U)"=0.0, "Stop Freq(Hz)"=0.0, "Ratio Val"=0.0, "ML val level name 2"="", "Use ML Val level? 2"=FALSE, "ML axis"=0, "Start Freq(Hz)"=0.0, "Step Resolution"=0, "Ratio"=0, "TabCtrl6"=enum."Master Tone", "unit 1"=0, "unit 2"=0} ("Value"), binary string=w667) -> (value=w638:T25)  [unwired: 1 in, 4 out]
              n164 = Unbundle By Name(w638) -> ("Level(U)"=w658:dbl, "Use ML Val level?"=w657:bool, "ML axis"=w656:u8, "ML val level name"=w655:string, "Start Freq(Hz)"=w654:dbl, "Stop Freq(Hz)"=w653:dbl, "Step Resolution"=w652:u16, "Steps (#)"=w651:i32, "Cycles/step (#)"=w650:u32, "Freq2(Hz)"=w649:dbl, "Level(U) 2"=w648:dbl, "Use ML Val level? 2"=w647:bool, "ML axis 2"=w646:u8, "ML val level name 2"=w645:string, "Diff Freq(Hz)"=w644:dbl, "Tone Type"=w643:u8, "Diff/Ratio"=w642:u8, "Ratio"=w641:u16, "Ratio Val"=w640:dbl, "Time/step (s)"=w639:dbl, "unit 1"=w635:u16, "unit 2"=w634:u16)
              n165 = Bundle By Name(cluster=w637, "Level(U)"=w658, "Use ML Val level?"=w657, "ML axis"=w656, "ML val level name"=w655, "Start Freq(Hz)"=w654, "Stop Freq(Hz)"=w653, "Step Resolution"=w652, "Steps (#)"=w651, "Cycles/step (#)"=w650, "Freq2(Hz)"=w649, "Level(U) 2"=w648, "Use ML Val level? 2"=w647, "ML axis"=w646, "ML val level name 2"=w645, "Diff Freq(Hz)"=w644, "Tone Type"=w643, "Diff/Ratio"=w642, "Ratio"=w641, "Ratio Val"=w640, "Time/step (s)"=w639, "unit 1"=w635, "unit 2"=w634) -> (w659:T7)
              n166 = property on="twotone" class="Clust (strict)"("Value"=w659) -> ()  [unwired: 2 in, 2 out]
              n167 = case shown="True" w657 {
                tunnel: w656 -> [_ w676]
                tunnel: w658 -> [w673 _]
                tunnel: [w673 w674] -> w661
                tunnel: w655 -> [_ w675]
                frame False {
                }
                frame True {
                  n168 = call "CRYGet Value from Curve Name.vi"("ML axis"=w676, "Level Name"=w675) -> ("Linear Value"=w674:dbl)  [unwired: 9 in]
                }
              }
              n169 = case shown="True" w647 {
                tunnel: w646 -> [_ w672]
                tunnel: w648 -> [w669 _]
                tunnel: [w669 w670] -> w660
                tunnel: w645 -> [_ w671]
                frame False {
                }
                frame True {
                  n170 = call "CRYGet Value from Curve Name.vi"("ML axis"=w672, "Level Name"=w671) -> ("Linear Value"=w670:dbl)  [unwired: 9 in]
                }
              }
              n171 = To Double Precision Float(number=w649) -> (double precision float=w663:dbl)
              n172 = Bundle By Name(cluster=w666, "Level Out"=w661, "Start Freq"=w654, "Stop Freq"=w653, "Resolution"=w652, "Steps"=w651, "Cycles"=w650, "Freq"=w663, "Start ampl"=w660, "Sweep type"=5, "Difference6"=w644, "Tone type6"=w643, "fix/ratio6"=w642, "Ratio6"=w641, "RatioFreq6"=w640, "Sweep time"=w639) -> (w665:T1)
            }
            frame "noise" {
              w679 = T9 {"Noise Type"=0, "Min Freq(Hz)"=20.0, "Max Freq(Hz)"=20000.0, "Level(U)"=1.0, "Duration(s)"=1.0, "ML val level name"="", "Use ML Val level?"=FALSE, "ML axis"=1, "unit"=0, "Start Freq Name"="", "Stop Freq Name"="", "Start Freq Axis"=0, "Stop Freq Axis"=0, "Start Freq Flag"="", "Stop Freq Flag"="", "Output Imp"=0.0, "Nominal Imp"=0.0, "V on DUT"=FALSE}  # noise
              n173 = Unflatten From String(type=T26 {"Noise Type"=0, "Min Freq(Hz)"=0.0, "Max Freq(Hz)"=0.0, "Level(U)"=0.0, "Duration(s)"=0.0, "ML val level name"="", "Use ML Val level?"=FALSE, "ML axis"=0, "unit"=0} ("Value"), binary string=w697) -> (value=w695:T26)  [unwired: 1 in, 4 out]
              n174 = Unbundle By Name(w695) -> ("Min Freq(Hz)"=w688:dbl, "Max Freq(Hz)"=w687:dbl, "Level(U)"=w686:dbl, "Duration(s)"=w685:dbl, "Noise Type"=w684:u8, "Use ML Val level?"=w683:bool, "ML axis"=w682:u8, "ML val level name"=w681:string, "unit"=w677:u16)
              n175 = Bundle By Name(cluster=w679, "Min Freq(Hz)"=w688, "Max Freq(Hz)"=w687, "Level(U)"=w686, "Duration(s)"=w685, "Noise Type"=w684, "Use ML Val level?"=w683, "ML axis"=w682, "ML val level name"=w681, "unit"=w677) -> (w680:T9)
              n176 = property on="noise" class="Clust (strict)"("Value"=w680) -> ()  [unwired: 2 in, 2 out]
              n177 = case shown="True" w683 {
                tunnel: w682 -> [_ w702]
                tunnel: w686 -> [w699 _]
                tunnel: [w699 w700] -> w689
                tunnel: w681 -> [_ w701]
                frame False {
                }
                frame True {
                  n178 = call "CRYGet Value from Curve Name.vi"("ML axis"=w702, "Level Name"=w701) -> ("Linear Value"=w700:dbl)  [unwired: 9 in]
                }
              }
              n179 = Bundle By Name(cluster=w696, "Level Out"=w689, "Start Freq"=w688, "Stop Freq"=w687, "Sweep type"=6, "Sweep time"=w685, "Tone type6"=w684, "Resolution"=u16 5, "Steps"=u32 1) -> (w694:T1)
            }
            frame "mltitone" {
              w705 = T8 {"Level(U)"=0.0, "Min Freq(Hz)"=0.0, "Max Freq(Hz)"=0.0, "Duration(s)"=0.0, "Freq Rounding"=FALSE, "Rounding Val"=5.0, "Profile"=0, "ML axis 2"=0, "ML val level name"="", "Use ML Val level?"=FALSE, "ML axis"=0, "Step Resolution"=0, "unit"=0, "Start Freq Name"="Calibration sens-out Left", "Stop Freq Name"="Calibration sens-out Left", "Start Freq Axis"=0, "Stop Freq Axis"=0, "Start Freq Flag"="", "Stop Freq Flag"="", "Output Imp"=0.0, "Nominal Imp"=0.0, "V on DUT"=FALSE}  # mltitone
              n180 = Unflatten From String(type=T27 {"Level(U)"=0.0, "Min Freq(Hz)"=0.0, "Max Freq(Hz)"=0.0, "Duration(s)"=0.0, "Freq Rounding"=FALSE, "Rounding Val"=0.0, "Profile"=0, "ML axis 2"=0, "ML val level name"="", "Use ML Val level?"=FALSE, "ML axis"=0, "Step Resolution"=0, "unit"=0} ("Value"), binary string=w725) -> (value=w724:T27)  [unwired: 1 in, 4 out]
              n181 = Unbundle By Name(w724) -> ("Level(U)"=w714:dbl, "Min Freq(Hz)"=w713:dbl, "Max Freq(Hz)"=w712:dbl, "Profile"=w711:i32, "Duration(s)"=w710:dbl, "Step Resolution"=w709:u16, "Use ML Val level?"=w708:bool, "ML axis"=w707:u8, "ML val level name"=w706:string, "unit"=w703:u16)
              n182 = Bundle By Name(cluster=w705, "Level(U)"=w714, "Min Freq(Hz)"=w713, "Max Freq(Hz)"=w712, "Profile"=w711, "Duration(s)"=w710, "Step Resolution"=w709, "Use ML Val level?"=w708, "ML axis"=w707, "ML val level name"=w706, "unit"=w703, "Freq Rounding"=FALSE, "Rounding Val"=0.0, "ML axis 2"=u8 0) -> (w715:T8)
              n183 = property on="mltitone" class="Clust (strict)"("Value"=w715) -> ()  [unwired: 2 in, 2 out]
              n184 = case shown="True" w708 {
                tunnel: w707 -> [_ w730]
                tunnel: w714 -> [w727 _]
                tunnel: [w727 w728] -> w719
                tunnel: w706 -> [_ w729]
                frame False {
                }
                frame True {
                  n185 = call "CRYGet Value from Curve Name.vi"("ML axis"=w730, "Level Name"=w729) -> ("Linear Value"=w728:dbl)  [unwired: 9 in]
                }
              }
              n186 = Bundle By Name(cluster=w723, "Level Out"=w719, "Start Freq"=w713, "Stop Freq"=w712, "Steps"=w711, "Sweep time"=w710, "Resolution"=w709, "Sweep type"=7) -> (w722:T1)
            }
          }
        }
        frame 4 {
          n187 = case shown="\"ampsw\"" w733 {
            tunnel: w737 -> [_ w762 w788 w813 w836 w862 w897 w927 w955]
            tunnel: [errorcluster {"status"=TRUE, "code"=0, "source"=""} ("error in (no error)") w761 w787 w812 w837 w863 w898 w928 w956] -> w736
            tunnel: w735 -> [_ w761 w787 w812 w837 w863 w898 w928 w956]
            tunnel: w731 -> [w739 w757 w785 w810 w834 w861 w896 w926 w953]
            tunnel: [w739 w759 w783 w808 w835 w860 w895 w924 w952] -> w734
            tunnel: ["" "Frequency Stepped Sweep" "Frequency Log Sweep" "Log Amplitude Sweep" "WAV" "DC Connect" "Two Tone" "Noise" "Multitone"] -> w732
            frame Default {
            }
            frame "fstepsw" {
              w741 = T30 {"Level(U)"=0.7071067811865476, "Start Freq(Hz)"=20000.0, "Stop Freq(Hz)"=20.0, "ML val level name"="Calibration sens-out Left", "Use ML Val level?"=FALSE, "ML axis"=0, "Steps (#)"=31, "Cycles/step(#)"=20, "Time/step (s)"=0.01, "Step Resolution"=0, "unit"=0, "Start Freq Name"="Calibration sens-out Left", "Stop Freq Name"="Calibration sens-out Left", "Start Freq Axis"=0, "Stop Freq Axis"=0, "Start Freq Flag"="", "Stop Freq Flag"=""}  # fstepsw
              w743 = T2 {"Level(U)"=0.7071067811865476, "Start Freq(Hz)"=20000.0, "Stop Freq(Hz)"=20.0, "ML val level name"="Calibration sens-out Left", "Use ML Val level?"=FALSE, "ML axis"=0, "Steps (#)"=31, "Cycles/step(#)"=20, "Time/step (s)"=0.01, "Step Resolution"=0, "unit"=0, "Start Freq Name"="Calibration sens-out Left", "Stop Freq Name"="Calibration sens-out Left", "Start Freq Axis"=0, "Stop Freq Axis"=0, "Start Freq Flag"="", "Stop Freq Flag"="", "Output Imp"=0.0, "Nominal Imp"=1.0, "V on DUT"=FALSE}  # fstepsw 4.0
              n188 = Unflatten From String(type=w741, binary string=w762) -> (value=w758:T30)  [unwired: 1 in, 4 out]
              n189 = Unbundle By Name(w758) -> ("Start Freq(Hz)"=w753:dbl, "Stop Freq(Hz)"=w752:dbl, "Steps (#)"=w751:i32, "Step Resolution"=w750:u16, "Cycles/step(#)"=w749:u32, "Time/step (s)"=w748:dbl, "Level(U)"=w747:dbl, "Use ML Val level?"=w746:bool, "ML axis"=w745:u8, "ML val level name"=w744:string, "unit"=w742:u16)
              n190 = Bundle By Name(cluster=w743, "Start Freq(Hz)"=w753, "Stop Freq(Hz)"=w752, "Steps (#)"=w751, "Step Resolution"=w750, "Cycles/step(#)"=w749, "Time/step (s)"=w748, "Level(U)"=w747, "Use ML Val level?"=w746, "ML axis"=w745, "ML val level name"=w744, "unit"=w742) -> (w754:T2)
              n191 = property on="fstepsw" class="Clust (strict)"("Value"=w754) -> ()  [unwired: 2 in, 2 out]
              n192 = case shown="True" w746 {
                tunnel: w745 -> [_ w766]
                tunnel: w747 -> [w763 _]
                tunnel: [w763 w764] -> w755
                tunnel: w744 -> [_ w765]
                frame False {
                }
                frame True {
                  n193 = call "CRYGet Value from Curve Name.vi"("ML axis"=w766, "Level Name"=w765) -> ("Linear Value"=w764:dbl)  [unwired: 9 in]
                }
              }
              n194 = Bundle By Name(cluster=w757, "Start Freq"=w753, "Stop Freq"=w752, "Resolution"=w750, "Steps"=w751, "Cycles"=w749, "Sweep type"=0, "Sweep time"=w748, "Level Out"=w755) -> (w759:T1)
            }
            frame "flogsw" {
              w767 = T31 {"Level(U)"=1.0, "Start Freq(Hz)"=100.0, "Stop Freq(Hz)"=6300.0, "Sweep Rate(s/dec)"=1.0, "Use ML Val level?"=FALSE, "ML val level name"="", "ML axis"=1, "TSR params"={"FSamp"=0.0, "FStart"=0.0, "FStop"=0.0, "NOffset"=0.0, "MStop"=0.0, "MStart"=0.0, "NHarm"=0.0, "Tsamp"=0.0, "Amplit"=0.0}, "unit"=0, "Start Freq Name"="Calibration sens-out Left", "Stop Freq Name"="Calibration sens-out Left", "Start Freq Axis"=0, "Stop Freq Axis"=0, "Start Freq Flag"="", "Stop Freq Flag"=""}  # flogsw
              w769 = T3 {"Level(U)"=1.0, "Start Freq(Hz)"=100.0, "Stop Freq(Hz)"=6300.0, "Sweep Rate(s/dec)"=1.0, "Use ML Val level?"=FALSE, "ML val level name"="", "ML axis"=1, "TSR params"={"FSamp"=0.0, "FStart"=0.0, "FStop"=0.0, "NOffset"=0.0, "MStop"=0.0, "MStart"=0.0, "NHarm"=0.0, "Tsamp"=0.0, "Amplit"=0.0}, "unit"=0, "Start Freq Name"="Calibration sens-out Left", "Stop Freq Name"="Calibration sens-out Left", "Start Freq Axis"=0, "Stop Freq Axis"=0, "Start Freq Flag"="", "Stop Freq Flag"="", "Output Imp"=0.0, "Nominal Imp"=1.0, "V on DUT"=FALSE}  # flogsw
              n195 = Unflatten From String(type=w767, binary string=w788) -> (value=w786:T31)  [unwired: 1 in, 4 out]
              n196 = Unbundle By Name(w786) -> ("Level(U)"=w777:dbl, "Start Freq(Hz)"=w776:dbl, "Stop Freq(Hz)"=w775:dbl, "Sweep Rate(s/dec)"=w774:dbl, "Use ML Val level?"=w773:bool, "ML axis"=w772:u8, "ML val level name"=w771:string, "TSR params"=w770:T29, "unit"=w768:u16)
              n197 = Bundle By Name(cluster=w769, "Level(U)"=w777, "Start Freq(Hz)"=w776, "Stop Freq(Hz)"=w775, "Sweep Rate(s/dec)"=w774, "Use ML Val level?"=w773, "ML axis"=w772, "ML val level name"=w771, "TSR params"=w770, "unit"=w768) -> (w778:T3)
              n198 = property on="flogsw" class="Clust (strict)"("Value"=w778) -> ()  [unwired: 2 in, 2 out]
              n199 = case shown="True" w773 {
                tunnel: w772 -> [_ w792]
                tunnel: w777 -> [w789 _]
                tunnel: [w789 w790] -> w779
                tunnel: w771 -> [_ w791]
                frame False {
                }
                frame True {
                  n200 = call "CRYGet Value from Curve Name.vi"("ML axis"=w792, "Level Name"=w791) -> ("Linear Value"=w790:dbl)  [unwired: 9 in]
                }
              }
              n201 = Bundle By Name(cluster=w785, "Level Out"=w779, "Start Freq"=w776, "Stop Freq"=w775, "Sweep type"=1, "Sweep time"=w774, "Resolution"=u16 5, "Steps"=u32 1) -> (w783:T1)
            }
            frame "ampsw" {
              w793 = T23 {"Freq(Hz)"=1000.0, "Steps (#)"=19, "Cycles(#)"=12, "Use ML Val freq?"=FALSE, "ML val freq name"="", "ML axis"=1, "Start Ampl(U)"=0.5, "Stop Ampl(U)"=1.0, "unit"=0}  # ampsw
              w795 = T4 {"Freq(Hz)"=1000.0, "Steps (#)"=19, "Cycles(#)"=12, "Use ML Val freq?"=FALSE, "ML val freq name"="", "ML axis"=1, "Start Ampl(U)"=0.5, "Stop Ampl(U)"=1.0, "unit"=0}  # ampsw
              n202 = Unflatten From String(type=w793, binary string=w813) -> (value=w811:T23)  [unwired: 1 in, 4 out]
              n203 = Unbundle By Name(w811) -> ("Freq(Hz)"=w803:dbl, "Steps (#)"=w802:i32, "Cycles(#)"=w801:u32, "Use ML Val freq?"=w800:bool, "ML axis"=w799:u8, "ML val freq name"=w798:string, "Start Ampl(U)"=w797:dbl, "Stop Ampl(U)"=w796:dbl, "unit"=w794:u16)
              n204 = Bundle By Name(cluster=w795, "Freq(Hz)"=w803, "Steps (#)"=w802, "Cycles(#)"=w801, "Use ML Val freq?"=w800, "ML axis"=w799, "ML val freq name"=w798, "Start Ampl(U)"=w797, "Stop Ampl(U)"=w796, "unit"=w794) -> (w804:T4)
              n205 = property on="ampsw" class="Clust (strict)"("Value"=w804) -> ()  [unwired: 2 in, 2 out]
              n206 = case shown="True" w800 {
                tunnel: w799 -> [_ w817]
                tunnel: w803 -> [w814 _]
                tunnel: [w814 w815] -> w805
                tunnel: w798 -> [_ w816]
                frame False {
                }
                frame True {
                  n207 = call "CRYGet Value from Curve Name.vi"("ML axis"=w817, "Level Name"=w816) -> ("Linear Value"=w815:dbl)  [unwired: 9 in]
                }
              }
              n208 = Bundle By Name(cluster=w810, "Steps"=w802, "Cycles"=w801, "Sweep type"=2, "Freq"=w805, "Start ampl"=w797, "Stop ampl"=w796, "Resolution"=u16 5) -> (w808:T1)
            }
            frame "wavefile" {
              w818 = T24 {"Level(U)"=0.0, "Wave Path"="", "ML axis"=1, "ML val level name"="", "Use ML Val level?"=FALSE, "wave info"="", "wave time"="", "Peak value4"=0.0, "RMS value4"=0.0, "wave channel"=0, "unit"=0}  # wavefile
              w820 = T5 {"Level(U)"=0.0, "Wave Path"="", "ML axis"=1, "ML val level name"="", "Use ML Val level?"=FALSE, "wave info"="", "wave time"="", "Peak value4"=0.0, "RMS value4"=0.0, "wave channel"=0, "unit"=0, "Output Imp"=0.0, "Nominal Imp"=1.0, "V on DUT"=FALSE}  # wavefile
              n209 = Unflatten From String(type=w818, binary string=w836) -> (value=w828:T24)  [unwired: 1 in, 4 out]
              n210 = Unbundle By Name(w828) -> ("Level(U)"=w826:dbl, "Wave Path"=w825:string, "Use ML Val level?"=w824:bool, "ML axis"=w823:u8, "ML val level name"=w822:string, "wave channel"=w821:u16, "unit"=w819:u16)
              n211 = Bundle By Name(cluster=w820, "Level(U)"=w826, "Wave Path"=w825, "Use ML Val level?"=w824, "ML axis"=w823, "ML val level name"=w822, "wave channel"=w821, "unit"=w819) -> (w827:T5)
              n212 = property on="wavefile" class="Clust (strict)"("Value"=w827) -> ()  [unwired: 2 in, 2 out]
              n213 = case shown="True" w824 {
                tunnel: w823 -> [_ w841]
                tunnel: w826 -> [w838 _]
                tunnel: [w838 w839] -> w829
                tunnel: w822 -> [_ w840]
                frame False {
                }
                frame True {
                  n214 = call "CRYGet Value from Curve Name.vi"("ML axis"=w841, "Level Name"=w840) -> ("Linear Value"=w839:dbl)  [unwired: 9 in]
                }
              }
              n215 = Bundle By Name(cluster=w834, "Level Out"=w829, "wav path"=w825, "Sweep type"=3, "Resolution"=u16 5, "Steps"=u32 1, "Tone type6"=w821) -> (w835:T1)
            }
            frame "dcconn" {
              w842 = T16 {"dc ctrl"=0, "dcmax I"=0, "dc polar"=0, "dc ctrl"=0, "Steps (#)"=19, "Time/step (s)"=0.05, "Start Ampl(U)"=1.0, "Stop Ampl(U)"=1.0, "Level(U)"=1.0, "Step Size"=1.0}  # dcconn
              w854 = T6 {"dc ctrl"=0, "dcmax I"=0, "dc polar"=0, "dc ctrl"=0, "Steps (#)"=19, "Time/step (s)"=0.05, "Start Ampl(U)"=1.0, "Stop Ampl(U)"=1.0, "Level(U)"=1.0, "Step Size"=1.0}  # dcconn
              n216 = Unflatten From String(type=w842, binary string=w862) -> (value=w859:T16)  [unwired: 1 in, 4 out]
              n217 = Unbundle By Name(w859) -> ("dc ctrl"=w852:u16, "dcmax I"=w851:u16, "dc polar"=w850:u16, "dc ctrl"=w849:u16, "Steps (#)"=w848:i32, "Time/step (s)"=w847:dbl, "Start Ampl(U)"=w846:dbl, "Stop Ampl(U)"=w845:dbl, "Level(U)"=w844:dbl, "Step Size"=w843:dbl)
              n218 = Bundle By Name(cluster=w854, "dc ctrl"=w852, "dcmax I"=w851, "dc polar"=w850, "dc ctrl"=w849, "Steps (#)"=w848, "Time/step (s)"=w847, "Start Ampl(U)"=w846, "Stop Ampl(U)"=w845, "Level(U)"=w844, "Step Size"=w843) -> (w853:T6)
              n219 = Bundle By Name(cluster=w861, "Sweep type"=4, "Start ampl"=w846, "Stop ampl"=w845, "Sweep time"=w847, "Resolution"=u16 5, "Steps"=u32 1) -> (w860:T1)
              n220 = property on="dcconn" class="Clust (strict)"("Value"=w853) -> ()  [unwired: 2 in, 2 out]
            }
            frame "twotone" {
              w864 = T32 {"Steps (#)"=19, "Tone Type"=0, "Freq2(Hz)"=1000.0, "Time/step (s)"=0.0, "Cycles/step (#)"=12, "ML val level name"="", "Use ML Val level?"=FALSE, "Level(U) 2"=1.0, "Diff Freq(Hz)"=100.0, "ML axis 2"=1, "Diff/Ratio"=0, "Level(U)"=1.0, "Stop Freq(Hz)"=100.0, "Ratio Val"=0.8, "ML val level name 2"="", "Use ML Val level? 2"=FALSE, "ML axis"=1, "Start Freq(Hz)"=6300.0, "Step Resolution"=0, "Ratio"=0, "TabCtrl6"=enum."Master Tone", "unit 1"=0, "unit 2"=0, "Start Freq Name"="", "Stop Freq Name"="", "Start Freq Axis"=0, "Stop Freq Axis"=0, "Start Freq Flag"="", "Stop Freq Flag"=""}  # twotone
              w867 = T7 {"Steps (#)"=19, "Tone Type"=0, "Freq2(Hz)"=1000.0, "Time/step (s)"=0.0, "Cycles/step (#)"=12, "ML val level name"="", "Use ML Val level?"=FALSE, "Level(U) 2"=1.0, "Diff Freq(Hz)"=100.0, "ML axis 2"=1, "Diff/Ratio"=0, "Level(U)"=1.0, "Stop Freq(Hz)"=100.0, "Ratio Val"=0.8, "ML val level name 2"="", "Use ML Val level? 2"=FALSE, "ML axis"=1, "Start Freq(Hz)"=6300.0, "Step Resolution"=0, "Ratio"=0, "TabCtrl6"=enum."Master Tone", "unit 1"=0, "unit 2"=0, "Start Freq Name"="", "Stop Freq Name"="", "Start Freq Axis"=0, "Stop Freq Axis"=0, "Start Freq Flag"="", "Stop Freq Flag"=""}  # twotone
              n221 = Unflatten From String(type=w864, binary string=w897) -> (value=w868:T32)  [unwired: 1 in, 4 out]
              n222 = Unbundle By Name(w868) -> ("Level(U)"=w888:dbl, "Use ML Val level?"=w887:bool, "ML axis"=w886:u8, "ML val level name"=w885:string, "Start Freq(Hz)"=w884:dbl, "Stop Freq(Hz)"=w883:dbl, "Step Resolution"=w882:u16, "Steps (#)"=w881:i32, "Cycles/step (#)"=w880:u32, "Freq2(Hz)"=w879:dbl, "Level(U) 2"=w878:dbl, "Use ML Val level? 2"=w877:bool, "ML axis 2"=w876:u8, "ML val level name 2"=w875:string, "Diff Freq(Hz)"=w874:dbl, "Tone Type"=w873:u8, "Diff/Ratio"=w872:u8, "Ratio"=w871:u16, "Ratio Val"=w870:dbl, "Time/step (s)"=w869:dbl, "unit 1"=w866:u16, "unit 2"=w865:u16)
              n223 = Bundle By Name(cluster=w867, "Level(U)"=w888, "Use ML Val level?"=w887, "ML axis"=w886, "ML val level name"=w885, "Start Freq(Hz)"=w884, "Stop Freq(Hz)"=w883, "Step Resolution"=w882, "Steps (#)"=w881, "Cycles/step (#)"=w880, "Freq2(Hz)"=w879, "Level(U) 2"=w878, "Use ML Val level? 2"=w877, "ML axis"=w876, "ML val level name 2"=w875, "Diff Freq(Hz)"=w874, "Tone Type"=w873, "Diff/Ratio"=w872, "Ratio"=w871, "Ratio Val"=w870, "Time/step (s)"=w869, "unit 1"=w866, "unit 2"=w865) -> (w889:T7)
              n224 = property on="twotone" class="Clust (strict)"("Value"=w889) -> ()  [unwired: 2 in, 2 out]
              n225 = case shown="True" w887 {
                tunnel: w886 -> [_ w906]
                tunnel: w888 -> [w903 _]
                tunnel: [w903 w904] -> w891
                tunnel: w885 -> [_ w905]
                frame False {
                }
                frame True {
                  n226 = call "CRYGet Value from Curve Name.vi"("ML axis"=w906, "Level Name"=w905) -> ("Linear Value"=w904:dbl)  [unwired: 9 in]
                }
              }
              n227 = case shown="True" w877 {
                tunnel: w876 -> [_ w902]
                tunnel: w878 -> [w899 _]
                tunnel: [w899 w900] -> w890
                tunnel: w875 -> [_ w901]
                frame False {
                }
                frame True {
                  n228 = call "CRYGet Value from Curve Name.vi"("ML axis"=w902, "Level Name"=w901) -> ("Linear Value"=w900:dbl)  [unwired: 9 in]
                }
              }
              n229 = To Double Precision Float(number=w879) -> (double precision float=w893:dbl)
              n230 = Bundle By Name(cluster=w896, "Level Out"=w891, "Start Freq"=w884, "Stop Freq"=w883, "Resolution"=w882, "Steps"=w881, "Cycles"=w880, "Freq"=w893, "Start ampl"=w890, "Sweep type"=5, "Difference6"=w874, "Tone type6"=w873, "fix/ratio6"=w872, "Ratio6"=w871, "RatioFreq6"=w870, "Sweep time"=w869) -> (w895:T1)
            }
            frame "noise" {
              w907 = T33 {"Noise Type"=0, "Min Freq(Hz)"=20.0, "Max Freq(Hz)"=20000.0, "Level(U)"=1.0, "Duration(s)"=1.0, "ML val level name"="", "Use ML Val level?"=FALSE, "ML axis"=1, "unit"=0, "Start Freq Name"="", "Stop Freq Name"="", "Start Freq Axis"=0, "Stop Freq Axis"=0, "Start Freq Flag"="", "Stop Freq Flag"=""}  # noise
              w909 = T9 {"Noise Type"=0, "Min Freq(Hz)"=20.0, "Max Freq(Hz)"=20000.0, "Level(U)"=1.0, "Duration(s)"=1.0, "ML val level name"="", "Use ML Val level?"=FALSE, "ML axis"=1, "unit"=0, "Start Freq Name"="", "Stop Freq Name"="", "Start Freq Axis"=0, "Stop Freq Axis"=0, "Start Freq Flag"="", "Stop Freq Flag"="", "Output Imp"=0.0, "Nominal Imp"=1.0, "V on DUT"=FALSE}  # noise
              n231 = Unflatten From String(type=w907, binary string=w927) -> (value=w925:T33)  [unwired: 1 in, 4 out]
              n232 = Unbundle By Name(w925) -> ("Min Freq(Hz)"=w918:dbl, "Max Freq(Hz)"=w917:dbl, "Level(U)"=w916:dbl, "Duration(s)"=w915:dbl, "Noise Type"=w914:u8, "Use ML Val level?"=w913:bool, "ML axis"=w912:u8, "ML val level name"=w911:string, "unit"=w908:u16)
              n233 = Bundle By Name(cluster=w909, "Min Freq(Hz)"=w918, "Max Freq(Hz)"=w917, "Level(U)"=w916, "Duration(s)"=w915, "Noise Type"=w914, "Use ML Val level?"=w913, "ML axis"=w912, "ML val level name"=w911, "unit"=w908) -> (w910:T9)
              n234 = property on="noise" class="Clust (strict)"("Value"=w910) -> ()  [unwired: 2 in, 2 out]
              n235 = case shown="True" w913 {
                tunnel: w912 -> [_ w932]
                tunnel: w916 -> [w929 _]
                tunnel: [w929 w930] -> w919
                tunnel: w911 -> [_ w931]
                frame False {
                }
                frame True {
                  n236 = call "CRYGet Value from Curve Name.vi"("ML axis"=w932, "Level Name"=w931) -> ("Linear Value"=w930:dbl)  [unwired: 9 in]
                }
              }
              n237 = Bundle By Name(cluster=w926, "Level Out"=w919, "Start Freq"=w918, "Stop Freq"=w917, "Sweep type"=6, "Sweep time"=w915, "Tone type6"=w914, "Resolution"=u16 5, "Steps"=u32 1) -> (w924:T1)
            }
            frame "mltitone" {
              w933 = T34 {"Level(U)"=0.0, "Min Freq(Hz)"=0.0, "Max Freq(Hz)"=0.0, "Duration(s)"=0.0, "Freq Rounding"=FALSE, "Rounding Val"=5.0, "Profile"=0, "ML axis 2"=0, "ML val level name"="", "Use ML Val level?"=FALSE, "ML axis"=0, "Step Resolution"=0, "unit"=0, "Start Freq Name"="Calibration sens-out Left", "Stop Freq Name"="Calibration sens-out Left", "Start Freq Axis"=0, "Stop Freq Axis"=0, "Start Freq Flag"="", "Stop Freq Flag"=""}  # mltitone
              w935 = T8 {"Level(U)"=0.0, "Min Freq(Hz)"=0.0, "Max Freq(Hz)"=0.0, "Duration(s)"=0.0, "Freq Rounding"=FALSE, "Rounding Val"=5.0, "Profile"=0, "ML axis 2"=0, "ML val level name"="", "Use ML Val level?"=FALSE, "ML axis"=0, "Step Resolution"=0, "unit"=0, "Start Freq Name"="Calibration sens-out Left", "Stop Freq Name"="Calibration sens-out Left", "Start Freq Axis"=0, "Stop Freq Axis"=0, "Start Freq Flag"="", "Stop Freq Flag"="", "Output Imp"=0.0, "Nominal Imp"=1.0, "V on DUT"=FALSE}  # mltitone
              n238 = Unflatten From String(type=w933, binary string=w955) -> (value=w954:T34)  [unwired: 1 in, 4 out]
              n239 = Unbundle By Name(w954) -> ("Level(U)"=w944:dbl, "Min Freq(Hz)"=w943:dbl, "Max Freq(Hz)"=w942:dbl, "Profile"=w941:i32, "Duration(s)"=w940:dbl, "Step Resolution"=w939:u16, "Use ML Val level?"=w938:bool, "ML axis"=w937:u8, "ML val level name"=w936:string, "unit"=w934:u16)
              n240 = Bundle By Name(cluster=w935, "Level(U)"=w944, "Min Freq(Hz)"=w943, "Max Freq(Hz)"=w942, "Profile"=w941, "Duration(s)"=w940, "Step Resolution"=w939, "Use ML Val level?"=w938, "ML axis"=w937, "ML val level name"=w936, "unit"=w934, "Freq Rounding"=FALSE, "Rounding Val"=0.0, "ML axis 2"=u8 0) -> (w945:T8)
              n241 = property on="mltitone" class="Clust (strict)"("Value"=w945) -> ()  [unwired: 2 in, 2 out]
              n242 = case shown="True" w938 {
                tunnel: w937 -> [_ w960]
                tunnel: w944 -> [w957 _]
                tunnel: [w957 w958] -> w949
                tunnel: w936 -> [_ w959]
                frame False {
                }
                frame True {
                  n243 = call "CRYGet Value from Curve Name.vi"("ML axis"=w960, "Level Name"=w959) -> ("Linear Value"=w958:dbl)  [unwired: 9 in]
                }
              }
              n244 = Bundle By Name(cluster=w953, "Level Out"=w949, "Start Freq"=w943, "Stop Freq"=w942, "Steps"=w941, "Sweep time"=w940, "Resolution"=w939, "Sweep type"=7) -> (w952:T1)
            }
          }
        }
        frame 5 {
          n245 = case shown="\"ampsw\"" w963 {
            selector: w963 -> [_ w979 w1014 _ _ _ w1112 w1156 w1192]
            tunnel: w967 -> [_ w978 w1013 w1059 w1082 w1108 w1113 w1155 w1191]
            tunnel: [errorcluster {"status"=TRUE, "code"=0, "source"=""} ("error in (no error)") w993 w1028 w1058 w1083 w1109 w1141 w1172 w1208] -> w966
            tunnel: w965 -> [_ w993 w1028 w1058 w1083 w1109 w1141 w1172 w1208]
            tunnel: w961 -> [w969 w987 w1027 w1057 w1080 w1107 w1140 w1171 w1207]
            tunnel: [w969 w989 w1025 w1051 w1081 w1106 w1139 w1170 w1206] -> w964
            tunnel: ["" "Frequency Stepped Sweep" "Frequency Log Sweep" "Log Amplitude Sweep" "WAV" "DC Connect" "Two Tone" "Noise" "Multitone"] -> w962
            frame Default {
            }
            frame "fstepsw" {
              w974 = T2 {"Level(U)"=1.0, "Start Freq(Hz)"=6300.0, "Stop Freq(Hz)"=100.0, "ML val level name"="", "Use ML Val level?"=FALSE, "ML axis"=1, "Steps (#)"=19, "Cycles/step(#)"=8, "Time/step (s)"=0.01, "Step Resolution"=0, "unit"=0, "Start Freq Name"="", "Stop Freq Name"="", "Start Freq Axis"=1, "Stop Freq Axis"=1, "Start Freq Flag"="", "Stop Freq Flag"="", "Output Imp"=0.0, "Nominal Imp"=1.0, "V on DUT"=FALSE}  # fstepsw
              n246 = Unflatten From String(type=w974, binary string=w978) -> (value=w975:T2)  [unwired: 1 in, 4 out]
              n247 = Unbundle By Name(w975) -> ("Steps (#)"=w992:i32, "Step Resolution"=w988:u16, "Cycles/step(#)"=w990:u32, "Time/step (s)"=w986:dbl, "Level(U)"=w982:dbl, "Use ML Val level?"=w980:bool, "ML axis"=w984:u8, "ML val level name"=w983:string, "Output Imp"=w972:dbl, "Nominal Imp"=w971:dbl, "V on DUT"=w973:bool)
              n248 = property on="fstepsw" class="Clust (strict)"("Value"=w975) -> ()  [unwired: 2 in, 2 out]
              n249 = call "CRYGet Freq From Flatten Data.vi"("Flattened Element Data"=w978, "Stimulus Type"=w979) -> ("Stop Freq(Hz)"=w976:dbl, "Start Freq(Hz)"=w977:dbl)  [unwired: 8 in]
              n250 = case shown="False" w980 {
                tunnel: w984 -> [_ w1006]
                tunnel: w982 -> [w998 _]
                tunnel: [w997 w1004] -> w981
                tunnel: w983 -> [_ w1005]
                tunnel: w973 -> [w996 _]
                tunnel: w972 -> [w995 _]
                tunnel: w971 -> [w994 _]
                frame False {
                  n251 = case shown="True" w996 {
                    tunnel: [w999 w1000] -> w997
                    tunnel: w998 -> [w999 w1003]
                    tunnel: w995 -> [_ w1002]
                    tunnel: w994 -> [_ w1001]
                    frame False {
                    }
                    frame True {
                      n252 = call "CRYCalc Voltage on DUT.vi"("VL"=w1003, "Rn"=w1001, "Ro"=w1002) -> ("Vo"=w1000:dbl)  [unwired: 8 in]
                    }
                  }
                }
                frame True {
                  n253 = call "CRYGet Value from Curve Name.vi"("ML axis"=w1006, "Level Name"=w1005) -> ("Linear Value"=w1004:dbl)  [unwired: 9 in]
                }
              }
              n254 = Bundle By Name(cluster=w987, "Start Freq"=w977, "Stop Freq"=w976, "Resolution"=w988, "Steps"=w992, "Cycles"=w990, "Sweep type"=0, "Sweep time"=w986, "Level Out"=w981) -> (w989:T1)
            }
            frame "flogsw" {
              w1010 = T3 {"Level(U)"=1.0, "Start Freq(Hz)"=100.0, "Stop Freq(Hz)"=6300.0, "Sweep Rate(s/dec)"=1.0, "Use ML Val level?"=FALSE, "ML val level name"="", "ML axis"=1, "TSR params"={"FSamp"=0.0, "FStart"=0.0, "FStop"=0.0, "NOffset"=0.0, "MStop"=0.0, "MStart"=0.0, "NHarm"=0.0, "Tsamp"=0.0, "Amplit"=0.0}, "unit"=0, "Start Freq Name"="Calibration sens-out Left", "Stop Freq Name"="Calibration sens-out Left", "Start Freq Axis"=0, "Stop Freq Axis"=0, "Start Freq Flag"="", "Stop Freq Flag"="", "Output Imp"=0.0, "Nominal Imp"=0.0, "V on DUT"=FALSE}  # flogsw
              n255 = Unflatten From String(type=w1010, binary string=w1013) -> (value=w1016:T3)  [unwired: 1 in, 4 out]
              n256 = Unbundle By Name(w1016) -> ("Level(U)"=w1015:dbl, "Sweep Rate(s/dec)"=w1024:dbl, "Use ML Val level?"=w1017:bool, "ML axis"=w1018:u8, "ML val level name"=w1019:string, "Output Imp"=w1008:dbl, "Nominal Imp"=w1007:dbl, "V on DUT"=w1009:bool)
              n257 = property on="flogsw" class="Clust (strict)"("Value"=w1016) -> ()  [unwired: 2 in, 2 out]
              n258 = case shown="True" w1017 {
                tunnel: w1018 -> [_ w1041]
                tunnel: w1015 -> [w1031 _]
                tunnel: [w1032 w1039] -> w1020
                tunnel: w1019 -> [_ w1040]
                tunnel: w1009 -> [w1033 _]
                tunnel: w1008 -> [w1030 _]
                tunnel: w1007 -> [w1029 _]
                frame False {
                  n259 = case shown="False" w1033 {
                    tunnel: [w1034 w1035] -> w1032
                    tunnel: w1031 -> [w1034 w1038]
                    tunnel: w1030 -> [_ w1037]
                    tunnel: w1029 -> [_ w1036]
                    frame False {
                    }
                    frame True {
                      n260 = call "CRYCalc Voltage on DUT.vi"("VL"=w1038, "Rn"=w1036, "Ro"=w1037) -> ("Vo"=w1035:dbl)  [unwired: 8 in]
                    }
                  }
                }
                frame True {
                  n261 = call "CRYGet Value from Curve Name.vi"("ML axis"=w1041, "Level Name"=w1040) -> ("Linear Value"=w1039:dbl)  [unwired: 9 in]
                }
              }
              n262 = call "CRYGet Freq From Flatten Data.vi"("Flattened Element Data"=w1013, "Stimulus Type"=w1014) -> ("Stop Freq(Hz)"=w1011:dbl, "Start Freq(Hz)"=w1012:dbl)  [unwired: 8 in]
              n263 = Bundle By Name(cluster=w1027, "Level Out"=w1020, "Start Freq"=w1012, "Stop Freq"=w1011, "Sweep type"=1, "Sweep time"=w1024, "Resolution"=u16 5, "Steps"=u32 1) -> (w1025:T1)
            }
            frame "ampsw" {
              w1043 = T4 {"Freq(Hz)"=1000.0, "Steps (#)"=19, "Cycles(#)"=12, "Use ML Val freq?"=FALSE, "ML val freq name"="", "ML axis"=1, "Start Ampl(U)"=0.5, "Stop Ampl(U)"=1.0, "unit"=0}  # ampsw
              n264 = Unflatten From String(type=w1043, binary string=w1059) -> (value=w1042:T4)  [unwired: 1 in, 4 out]
              n265 = Unbundle By Name(w1042) -> ("Freq(Hz)"=w1045:dbl, "Steps (#)"=w1052:i32, "Cycles(#)"=w1053:u32, "Use ML Val freq?"=w1048:bool, "ML axis"=w1047:u8, "ML val freq name"=w1046:string, "Start Ampl(U)"=w1055:dbl, "Stop Ampl(U)"=w1054:dbl)
              n266 = property on="ampsw" class="Clust (strict)"("Value"=w1042) -> ()  [unwired: 2 in, 2 out]
              n267 = case shown="False" w1048 {
                tunnel: w1047 -> [_ w1063]
                tunnel: w1045 -> [w1060 _]
                tunnel: [w1060 w1061] -> w1044
                tunnel: w1046 -> [_ w1062]
                frame False {
                }
                frame True {
                  n268 = call "CRYGet Value from Curve Name.vi"("ML axis"=w1063, "Level Name"=w1062) -> ("Linear Value"=w1061:dbl)  [unwired: 9 in]
                }
              }
              n269 = Bundle By Name(cluster=w1057, "Steps"=w1052, "Cycles"=w1053, "Sweep type"=2, "Freq"=w1044, "Start ampl"=w1055, "Stop ampl"=w1054, "Resolution"=u16 5) -> (w1051:T1)
            }
            frame "wavefile" {
              w1067 = T5 {"Level(U)"=0.0, "Wave Path"="", "ML axis"=1, "ML val level name"="", "Use ML Val level?"=FALSE, "wave info"="", "wave time"="", "Peak value4"=0.0, "RMS value4"=0.0, "wave channel"=0, "unit"=0, "Output Imp"=0.0, "Nominal Imp"=0.0, "V on DUT"=FALSE}  # wavefile
              n270 = Unflatten From String(type=w1067, binary string=w1082) -> (value=w1068:T5)  [unwired: 1 in, 4 out]
              n271 = Unbundle By Name(w1068) -> ("Level(U)"=w1074:dbl, "Wave Path"=w1079:string, "Use ML Val level?"=w1073:bool, "ML axis"=w1071:u8, "ML val level name"=w1070:string, "wave channel"=w1069:u16, "Output Imp"=w1066:dbl, "Nominal Imp"=w1065:dbl, "V on DUT"=w1064:bool)
              n272 = property on="wavefile" class="Clust (strict)"("Value"=w1068) -> ()  [unwired: 2 in, 2 out]
              n273 = case shown="False" w1073 {
                tunnel: w1071 -> [_ w1096]
                tunnel: w1074 -> [w1088 _]
                tunnel: [w1087 w1094] -> w1072
                tunnel: w1070 -> [_ w1095]
                tunnel: w1066 -> [w1086 _]
                tunnel: w1065 -> [w1085 _]
                tunnel: w1064 -> [w1084 _]
                frame False {
                  n274 = case shown="True" w1084 {
                    tunnel: [w1089 w1090] -> w1087
                    tunnel: w1088 -> [w1089 w1093]
                    tunnel: w1086 -> [_ w1092]
                    tunnel: w1085 -> [_ w1091]
                    frame False {
                    }
                    frame True {
                      n275 = call "CRYCalc Voltage on DUT.vi"("VL"=w1093, "Rn"=w1091, "Ro"=w1092) -> ("Vo"=w1090:dbl)  [unwired: 8 in]
                    }
                  }
                }
                frame True {
                  n276 = call "CRYGet Value from Curve Name.vi"("ML axis"=w1096, "Level Name"=w1095) -> ("Linear Value"=w1094:dbl)  [unwired: 9 in]
                }
              }
              n277 = Bundle By Name(cluster=w1080, "Level Out"=w1072, "wav path"=w1079, "Sweep type"=3, "Resolution"=u16 5, "Steps"=u32 1, "Tone type6"=w1069) -> (w1081:T1)
            }
            frame "dcconn" {
              w1097 = T6 {"dc ctrl"=0, "dcmax I"=0, "dc polar"=0, "dc ctrl"=0, "Steps (#)"=19, "Time/step (s)"=0.05, "Start Ampl(U)"=1.0, "Stop Ampl(U)"=1.0, "Level(U)"=1.0, "Step Size"=1.0}  # dcconn
              n278 = Unflatten From String(type=w1097, binary string=w1108) -> (value=w1098:T6)  [unwired: 1 in, 4 out]
              n279 = property on="dcconn" class="Clust (strict)"("Value"=w1098) -> ()  [unwired: 2 in, 2 out]
              n280 = Unbundle By Name(w1098) -> ("Time/step (s)"=w1105:dbl, "Start Ampl(U)"=w1104:dbl, "Stop Ampl(U)"=w1103:dbl)
              n281 = Bundle By Name(cluster=w1107, "Sweep type"=4, "Start ampl"=w1104, "Stop ampl"=w1103, "Sweep time"=w1105, "Resolution"=u16 5, "Steps"=u32 1) -> (w1106:T1)
            }
            frame "twotone" {
              w1114 = T7 {"Steps (#)"=19, "Tone Type"=0, "Freq2(Hz)"=1000.0, "Time/step (s)"=0.0, "Cycles/step (#)"=12, "ML val level name"="", "Use ML Val level?"=FALSE, "Level(U) 2"=1.0, "Diff Freq(Hz)"=100.0, "ML axis 2"=1, "Diff/Ratio"=0, "Level(U)"=1.0, "Stop Freq(Hz)"=100.0, "Ratio Val"=0.8, "ML val level name 2"="", "Use ML Val level? 2"=FALSE, "ML axis"=1, "Start Freq(Hz)"=6300.0, "Step Resolution"=0, "Ratio"=0, "TabCtrl6"=enum."Master Tone", "unit 1"=0, "unit 2"=0, "Start Freq Name"="", "Stop Freq Name"="", "Start Freq Axis"=0, "Stop Freq Axis"=0, "Start Freq Flag"="", "Stop Freq Flag"=""}  # twotone
              n282 = Unflatten From String(type=w1114, binary string=w1113) -> (value=w1115:T7)  [unwired: 1 in, 4 out]
              n283 = Unbundle By Name(w1115) -> ("Level(U)"=w1124:dbl, "Use ML Val level?"=w1125:bool, "ML axis"=w1123:u8, "ML val level name"=w1122:string, "Step Resolution"=w1137:u16, "Steps (#)"=w1136:i32, "Cycles/step (#)"=w1135:u32, "Freq2(Hz)"=w1134:dbl, "Level(U) 2"=w1121:dbl, "Use ML Val level? 2"=w1120:bool, "ML axis 2"=w1119:u8, "ML val level name 2"=w1118:string, "Diff Freq(Hz)"=w1132:dbl, "Tone Type"=w1131:u8, "Diff/Ratio"=w1130:u8, "Ratio"=w1129:u16, "Ratio Val"=w1128:dbl, "Time/step (s)"=w1127:dbl)
              n284 = property on="twotone" class="Clust (strict)"("Value"=w1115) -> ()  [unwired: 2 in, 2 out]
              n285 = case shown="True" w1125 {
                tunnel: w1123 -> [_ w1149]
                tunnel: w1124 -> [w1146 _]
                tunnel: [w1146 w1147] -> w1117
                tunnel: w1122 -> [_ w1148]
                frame False {
                }
                frame True {
                  n286 = call "CRYGet Value from Curve Name.vi"("ML axis"=w1149, "Level Name"=w1148) -> ("Linear Value"=w1147:dbl)  [unwired: 9 in]
                }
              }
              n287 = case shown="True" w1120 {
                tunnel: w1119 -> [_ w1145]
                tunnel: w1121 -> [w1142 _]
                tunnel: [w1142 w1143] -> w1116
                tunnel: w1118 -> [_ w1144]
                frame False {
                }
                frame True {
                  n288 = call "CRYGet Value from Curve Name.vi"("ML axis"=w1145, "Level Name"=w1144) -> ("Linear Value"=w1143:dbl)  [unwired: 9 in]
                }
              }
              n289 = call "CRYGet Freq From Flatten Data.vi"("Flattened Element Data"=w1113, "Stimulus Type"=w1112) -> ("Stop Freq(Hz)"=w1110:dbl, "Start Freq(Hz)"=w1111:dbl)  [unwired: 8 in]
              n290 = To Double Precision Float(number=w1134) -> (double precision float=w1133:dbl)
              n291 = Bundle By Name(cluster=w1140, "Level Out"=w1117, "Start Freq"=w1111, "Stop Freq"=w1110, "Resolution"=w1137, "Steps"=w1136, "Cycles"=w1135, "Freq"=w1133, "Start ampl"=w1116, "Sweep type"=5, "Difference6"=w1132, "Tone type6"=w1131, "fix/ratio6"=w1130, "Ratio6"=w1129, "RatioFreq6"=w1128, "Sweep time"=w1127) -> (w1139:T1)
            }
            frame "noise" {
              w1157 = T9 {"Noise Type"=0, "Min Freq(Hz)"=20.0, "Max Freq(Hz)"=20000.0, "Level(U)"=1.0, "Duration(s)"=1.0, "ML val level name"="", "Use ML Val level?"=FALSE, "ML axis"=1, "unit"=0, "Start Freq Name"="", "Stop Freq Name"="", "Start Freq Axis"=0, "Stop Freq Axis"=0, "Start Freq Flag"="", "Stop Freq Flag"="", "Output Imp"=0.0, "Nominal Imp"=0.0, "V on DUT"=FALSE}  # noise
              n292 = Unflatten From String(type=w1157, binary string=w1155) -> (value=w1158:T9)  [unwired: 1 in, 4 out]
              n293 = Unbundle By Name(w1158) -> ("Level(U)"=w1162:dbl, "Duration(s)"=w1168:dbl, "Noise Type"=w1164:u8, "Use ML Val level?"=w1161:bool, "ML axis"=w1160:u8, "ML val level name"=w1159:string, "Output Imp"=w1152:dbl, "Nominal Imp"=w1151:dbl, "V on DUT"=w1150:bool)
              n294 = property on="noise" class="Clust (strict)"("Value"=w1158) -> ()  [unwired: 2 in, 2 out]
              n295 = case shown="False" w1161 {
                tunnel: w1160 -> [_ w1185]
                tunnel: w1162 -> [w1177 _]
                tunnel: [w1176 w1183] -> w1163
                tunnel: w1159 -> [_ w1184]
                tunnel: w1152 -> [w1175 _]
                tunnel: w1151 -> [w1174 _]
                tunnel: w1150 -> [w1173 _]
                frame False {
                  n296 = case shown="True" w1173 {
                    tunnel: [w1178 w1179] -> w1176
                    tunnel: w1177 -> [w1178 w1182]
                    tunnel: w1175 -> [_ w1181]
                    tunnel: w1174 -> [_ w1180]
                    frame False {
                    }
                    frame True {
                      n297 = call "CRYCalc Voltage on DUT.vi"("VL"=w1182, "Rn"=w1180, "Ro"=w1181) -> ("Vo"=w1179:dbl)  [unwired: 8 in]
                    }
                  }
                }
                frame True {
                  n298 = call "CRYGet Value from Curve Name.vi"("ML axis"=w1185, "Level Name"=w1184) -> ("Linear Value"=w1183:dbl)  [unwired: 9 in]
                }
              }
              n299 = call "CRYGet Freq From Flatten Data.vi"("Flattened Element Data"=w1155, "Stimulus Type"=w1156) -> ("Stop Freq(Hz)"=w1153:dbl, "Start Freq(Hz)"=w1154:dbl)  [unwired: 8 in]
              n300 = Bundle By Name(cluster=w1171, "Level Out"=w1163, "Start Freq"=w1154, "Stop Freq"=w1153, "Sweep type"=6, "Sweep time"=w1168, "Tone type6"=w1164, "Resolution"=u16 5, "Steps"=u32 1) -> (w1170:T1)
            }
            frame "mltitone" {
              w1194 = T8 {"Level(U)"=0.0, "Min Freq(Hz)"=0.0, "Max Freq(Hz)"=0.0, "Duration(s)"=0.0, "Freq Rounding"=FALSE, "Rounding Val"=5.0, "Profile"=0, "ML axis 2"=0, "ML val level name"="", "Use ML Val level?"=FALSE, "ML axis"=0, "Step Resolution"=0, "unit"=0, "Start Freq Name"="Calibration sens-out Left", "Stop Freq Name"="Calibration sens-out Left", "Start Freq Axis"=0, "Stop Freq Axis"=0, "Start Freq Flag"="", "Stop Freq Flag"="", "Output Imp"=0.0, "Nominal Imp"=0.0, "V on DUT"=FALSE}  # mltitone
              n301 = Unflatten From String(type=w1194, binary string=w1191) -> (value=w1196:T8)  [unwired: 1 in, 4 out]
              n302 = Unbundle By Name(w1196) -> ("Level(U)"=w1193:dbl, "Profile"=w1205:i32, "Duration(s)"=w1204:dbl, "Step Resolution"=w1203:u16, "Use ML Val level?"=w1199:bool, "ML axis"=w1198:u8, "ML val level name"=w1197:string, "unit"=w1195:u16, "Output Imp"=w1187:dbl, "Nominal Imp"=w1186:dbl, "V on DUT"=w1188:bool)
              n303 = property on="mltitone" class="Clust (strict)"("Value"=w1196) -> ()  [unwired: 2 in, 2 out]
              n304 = call "CRYGet Freq From Flatten Data.vi"("Flattened Element Data"=w1191, "Stimulus Type"=w1192) -> ("Stop Freq(Hz)"=w1189:dbl, "Start Freq(Hz)"=w1190:dbl)  [unwired: 8 in]
              n305 = case shown="False" w1199 {
                tunnel: w1198 -> [_ w1221]
                tunnel: w1193 -> [w1213 _]
                tunnel: [w1211 w1219] -> w1200
                tunnel: w1197 -> [_ w1220]
                tunnel: w1188 -> [w1212 _]
                tunnel: w1187 -> [w1210 _]
                tunnel: w1186 -> [w1209 _]
                frame False {
                  n306 = case shown="True" w1212 {
                    tunnel: [w1214 w1215] -> w1211
                    tunnel: w1213 -> [w1214 w1218]
                    tunnel: w1210 -> [_ w1217]
                    tunnel: w1209 -> [_ w1216]
                    frame False {
                    }
                    frame True {
                      n307 = call "CRYCalc Voltage on DUT.vi"("VL"=w1218, "Rn"=w1216, "Ro"=w1217) -> ("Vo"=w1215:dbl)  [unwired: 8 in]
                    }
                  }
                }
                frame True {
                  n308 = call "CRYGet Value from Curve Name.vi"("ML axis"=w1221, "Level Name"=w1220) -> ("Linear Value"=w1219:dbl)  [unwired: 9 in]
                }
              }
              n309 = Bundle By Name(cluster=w1207, "Level Out"=w1200, "Start Freq"=w1190, "Stop Freq"=w1189, "Steps"=w1205, "Sweep time"=w1204, "Resolution"=w1203, "Sweep type"=7, "Ratio6"=w1195) -> (w1206:T1)
            }
          }
        }
      }
    }
  }
  "error out" <- w6
  "Stimulus Para" <- w1
  "Type Name" <- w3
  n310 = Bundle("Unflatten Stimulus Element setup"=w7, w9, "unsigned byte array[2]"=w8) -> (→"Header of common":T35)  [unwired: 1 out]
